vi "(150M)art联动采集V4.9(新增双行扫描模块).vi"() -> ()   [LabVIEW 2016]
uses:
  <vilib>/Utility/file.llb/Write Delimited Spreadsheet (DBL).vi
  E:/PCI8552B/Driver/INF/Win32&Win64/amd64/PCI8552B_32.dll
  <vilib>/Utility/file.llb/Read Delimited Spreadsheet (I64).vi
  <vilib>/Instr/_visa.llb/VISA Configure Serial Port (Instr).vi
panel:
  out "量程选择":i32(ring)=1 items=["±1000mV", "±5000mV"]
  out "待读取数据长度":i32
  in  "单行？":enum32{"单行", "双行"}(radio)
  in  "色码表导入":path=path "C:/Users/H301/Desktop/art闭环扫描程序/色码表/色码表（彩色2）.txt" caption="（色码表导入）"
  out "水平进度条":u8(slide) scale=0.0..100.0
  out "x+y 3":dbl=3.0
  in  "分层图查看":bool
  in  "hDevice 2":i32
  in  "逐行扫描":bool
  in  "定位模式":bool
  in  "X终点":dbl
  in  "Y终点":dbl
  in  "高级设置":bool
  in  "Y轴回零速度":dbl=15000.0
  in  "X轴回零速度":dbl=15000.0
  in  "细分设置":dbl=8.0
  in  "等待时间":u32=40
  in  "文件保存":path=path "C:/Users/H301/Desktop/art采集实验数据" caption="保存路径"
  out "已用时（s）":dbl format="%<%H:%M:%S>t"
  out "error out":errorcluster caption="错误输出"
  in  "退出扫描(Esc)":bool
  in  "N_Length":i32=8000000
  out "M_Length":i32
  out "hDevice":i32=241832032
  out "毫秒计时值":u32=3586537
  out "数组":dbl[][](array[numeric])=[[58819.77200735986, 88200.32943600747]]
  out "强度图":dbl[][](graph)=[[58819.77200735986, 88200.32943600747]]
  out "judge":dbl
  out "Xloop":dbl
  out "幅频谱":dbl[](graph)
  out "时域谱":dbl[](graph)
  out "错误输出":errorcluster
  in  "启动":bool
  in  "逐点扫描":bool
  in  "X归零":bool
  in  "Y归零":bool
  in  "Y起点":dbl
  in  "Y轴速度":dbl=9000.0
  in  "X轴速度":dbl=9000.0
  out "电机状态":bool
  in  "电机端口":refnum<visa-resource-name>="COM6"
  out "Yloop":dbl=1.0
  out "X扫描范围":dbl=150.0
  out "Y扫描范围":dbl=75.0
  out "Y序":i32
  in  "X起点":dbl
  out "Y(mm)":dbl
  out "x+y 2":dbl=3.0
  in  "Y:":dbl=1.0
  in  "精度":dbl=0.001
  in  "电机急停":bool
  out "X（mm）":dbl
  out "x+y":dbl=1.0
  in  "X:":dbl=1.0
  # "实时坐标"
  # "时域谱"
  # "频域谱"
  # "归零"
  # "扫描区域"
  # "扫描步进(mm)"
  # "X:"
  # "~"
  # "Y:"
  # "~"
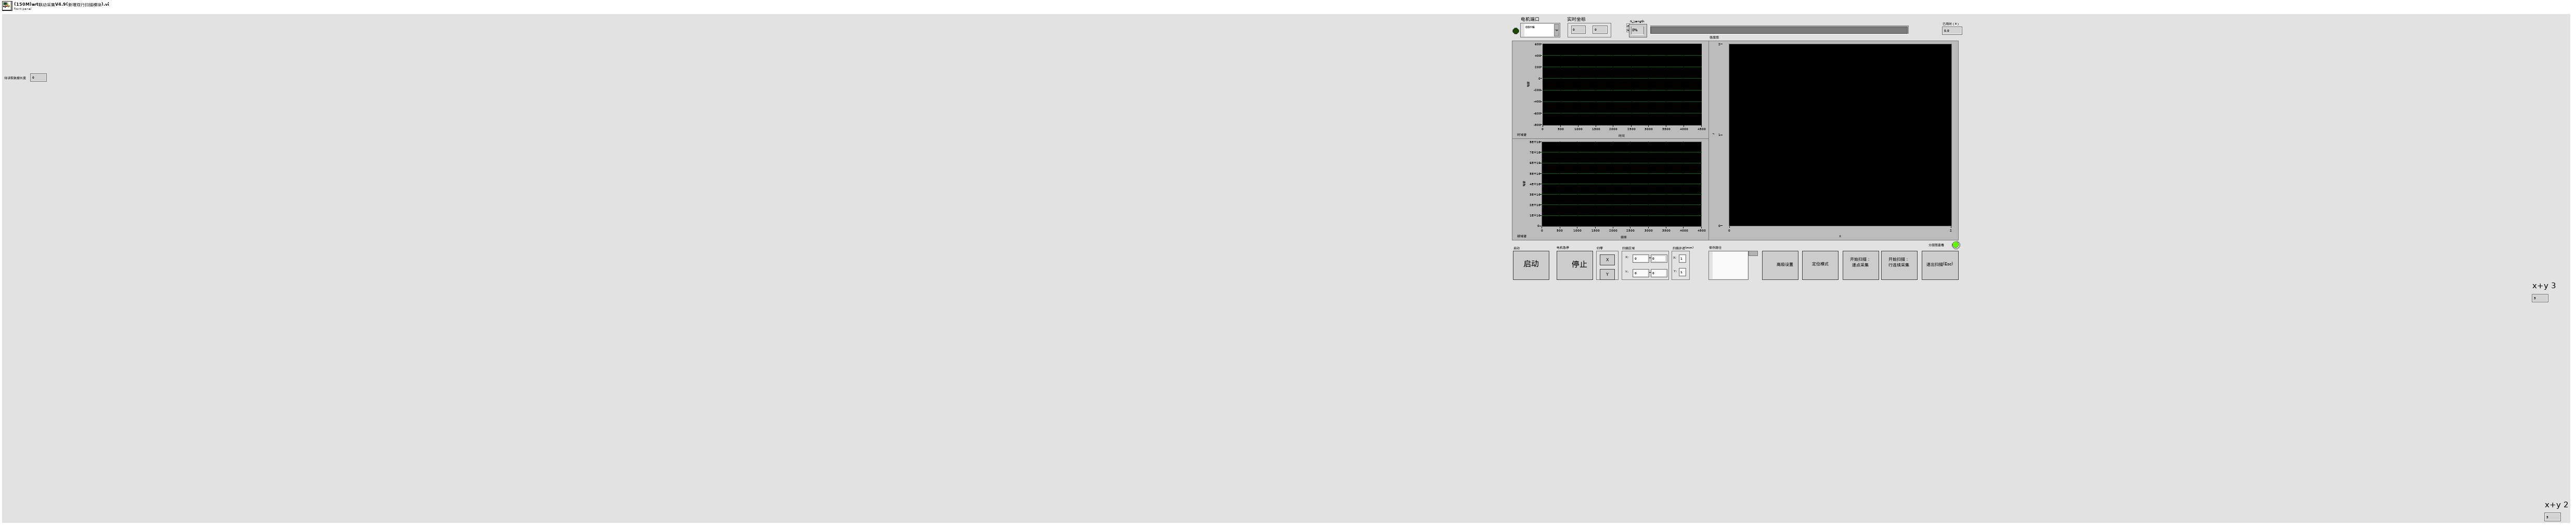
[diagram p1: front panel]
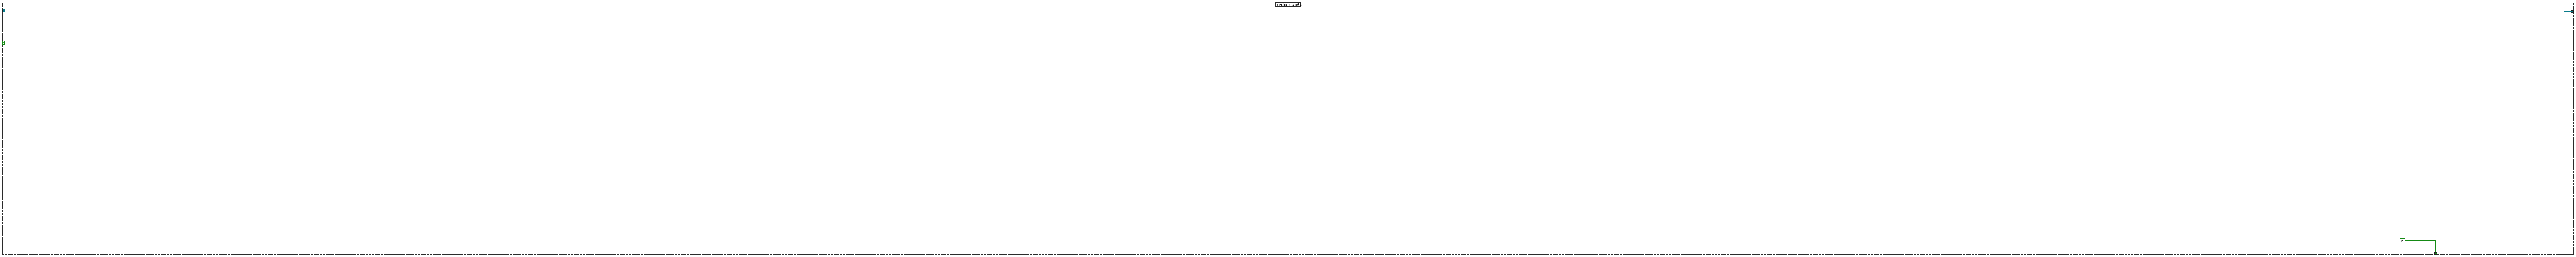
[diagram p3: hidden frame]
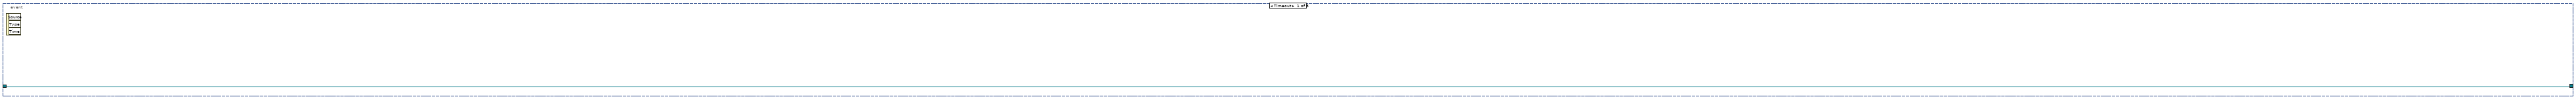
[diagram p4: hidden frame]
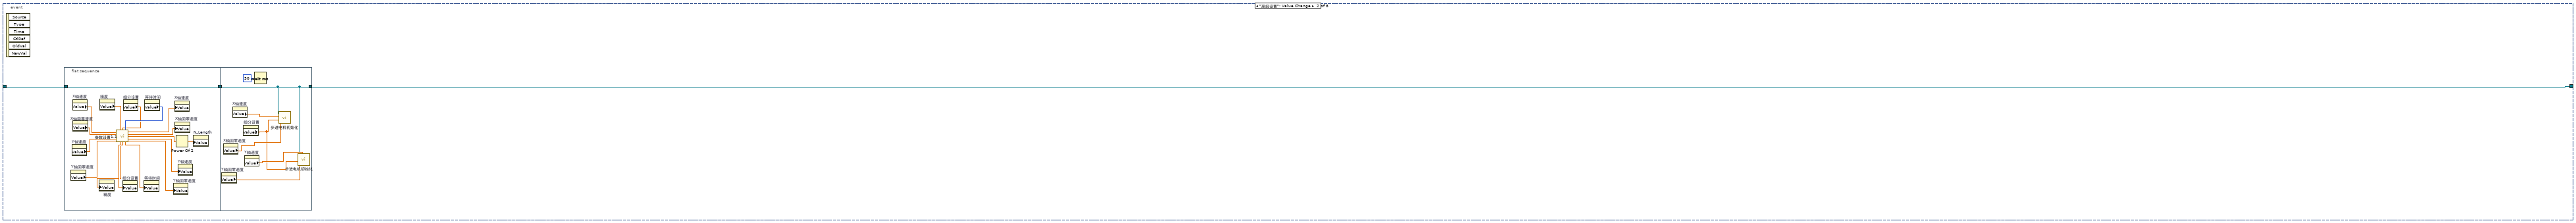
[diagram p5: hidden frame]
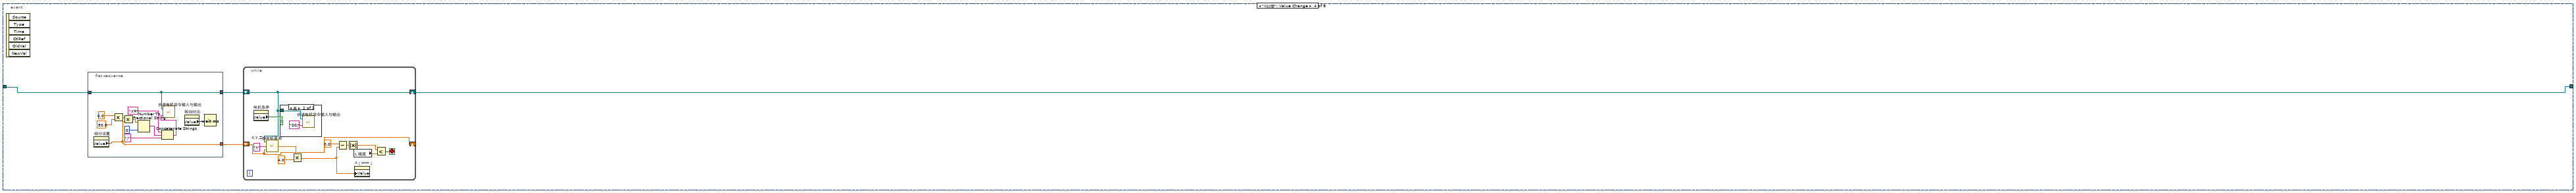
[diagram p6: hidden frame]
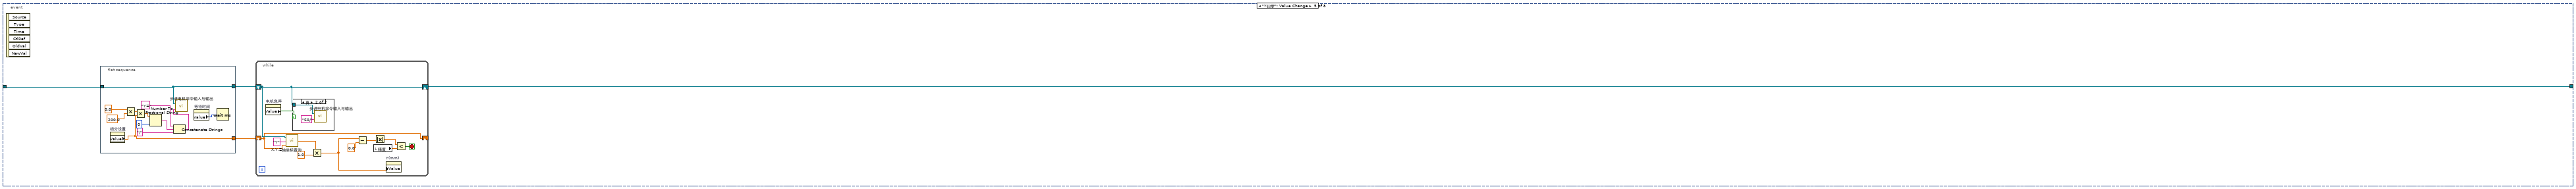
[diagram p8: hidden frame]
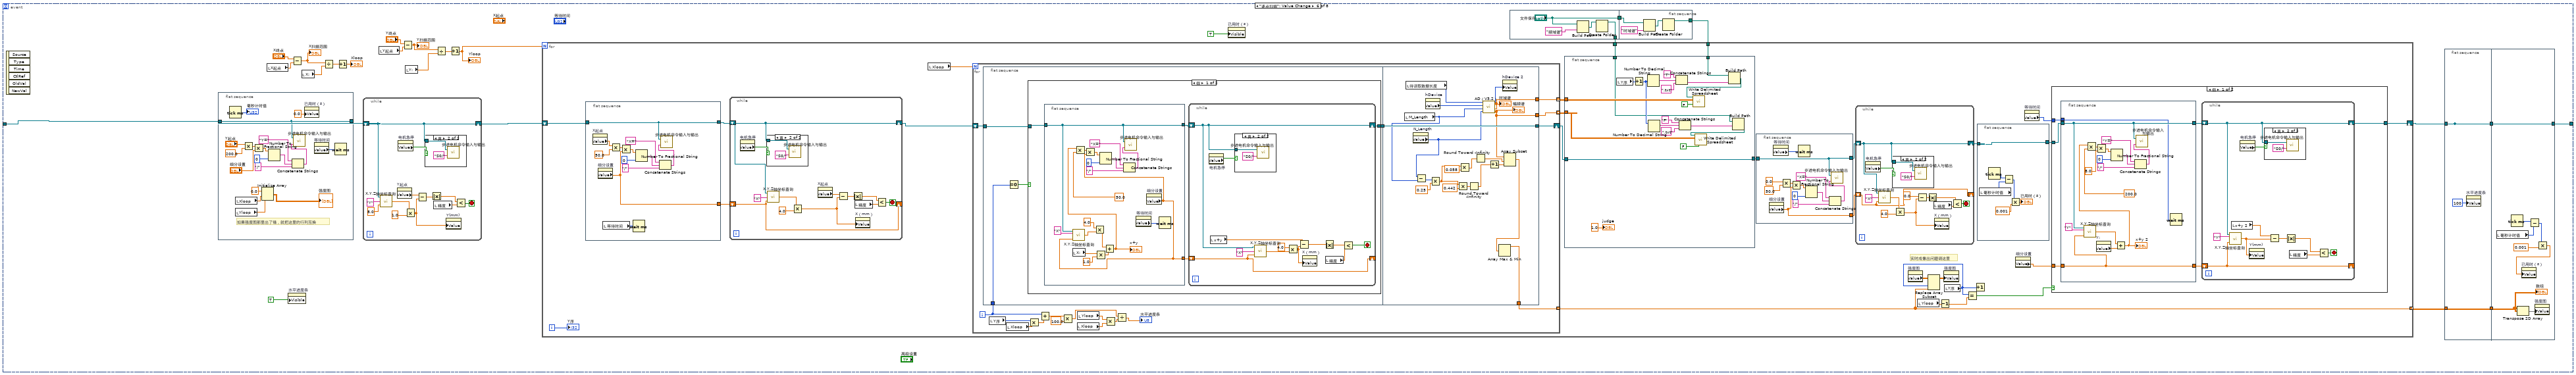
[diagram p10: hidden frame]
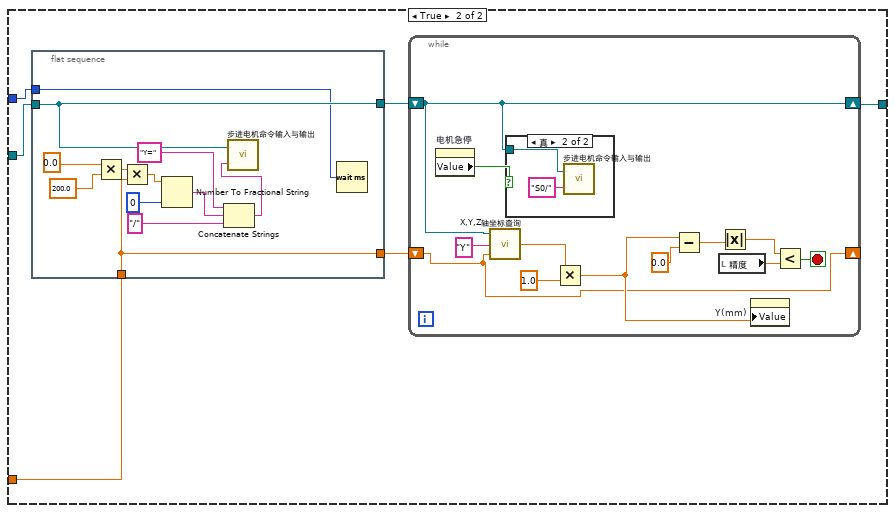
[diagram p15: hidden frame]
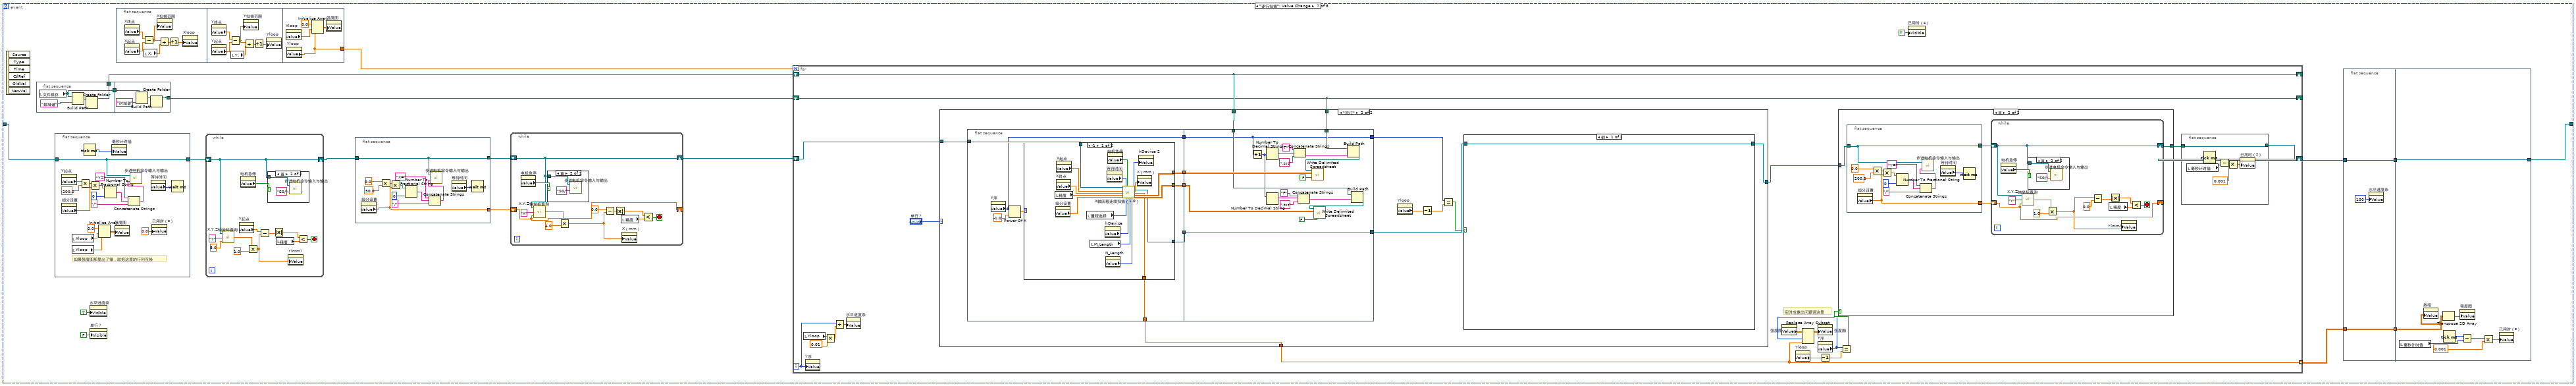
[diagram p19: hidden frame]
diagram:
  n1 = call-poly <vilib>:"Read Delimited Spreadsheet.vi"("file path (dialog if empty)"="色码表导入") -> ("first row"=w2:i64[])  [unwired: 9 in, 5 out]
  n2 = property on="强度图" class="IntGraph (严格)"("Color Table"=w2) -> ()  [unwired: 2 in, 2 out]
  n3 = property on="水平进度条" class="Slide (严格)"("Visible"=FALSE ("可见")) -> ()  [unwired: 2 in, 2 out]
  n4 = property on="单行？" class="RadioBtnsControl (严格)"("Visible"=TRUE ("可见")) -> ()  [unwired: 2 in, 2 out]
  n5 = while {
    stop <- w8 stop-if-true
    n6 = case shown="假" "启动" {
      tunnel: [FALSE ("ESC") w48] -> w8
      frame False {
      }
      frame True {
        w15 = 0  # M
        w25 = 1 items=["交流", "直流"]  # 耦合
        w23 = 1 items=["±1000mV", "±5000mV"]  # 量程选择
        w27 = TRUE  # 通道使能
        w21 = 20000000  # 采集频率
        w32 = 0 items=["中间触发", "后触发", "预触发", "硬件延时触发"]  # 触发模式
        w30 = 0 items=["通道0", "通道1"]  # ATR通道
        w41 = 0 items=["软件触发", "DTR作为触发源", "ATR作为触发源", "Trigger信号触发"]  # 触发源
        w40 = 0 items=["下降沿触发", "上升沿触发", "上下边沿均触发", ""]  # 触发方向
        w39 = 0  # 触发电平
        w24 = 1  # 触发次数
        w37 = 0 items=["TRIG0", "TRIG1", "TRIG2", "TRIG3"]  # 时钟输入输出源
        w38 = 0 items=["内时钟源", "主卡10M时钟源", "外部时钟"]  # 时钟源选择
        w61 = u16 0 items=["无", "XON/XOFF", "RTS/CTS", "XON/XOFF & RTS/CTS", "DTR/DSR", "XON/XOFF & DTR/DSR"] ("flow control (0:none)")
        w62 = u16 10 items=["1.0"=10, "1.5"=15, "2.0"=20] ("stop bits (10: 1 bit)")
        n7 = Boolean To (0,1)(Boolean=w27) -> (0, 1=w34:i16)
        n8 = Boolean To (0,1)(Boolean=FALSE ("主设备使能")) -> (0, 1=w35:i16)
        n9 = To Long Integer(number=w34) -> (32bit integer=w26:i32)
        n10 = To Long Integer(number=w35) -> (32bit integer=w36:i32)
        n11 = call-poly "VISA Configure Serial Port"("VISA resource name"="电机端口", "baud rate (9600)"=u32 9600, "data bits (8)"=u16 8, "parity (0:none)"=enum16{"None", "Odd", "Even", "Mark", "Space"}."None", "stop bits (10: 1 bit)"=w62, "flow control (0:none)"=w61) -> ("VISA resource name out"=w53:refnum<visa-resource-name>, "error out"=→"error out":errorcluster)  [unwired: 1 in, 7 out]
        n12 = Build Array(w26, w26) -> (w22:i32[])
        n13 = Build Array(w23, w23) -> (w31:i32[])
        n14 = Build Array(w25, w25) -> (w42:i32[])
        n15 = property on="细分设置" class="DigNum (严格)"() -> ("Value"=w47:dbl)  [unwired: 2 in, 2 out]
        n16 = Add Array Elements(numeric array=w22) -> (sum=w17:i32)
        n17 = Build Array (concatenate)(w22, w21, w31, w42, w15, "N_Length", w32, w30, w41, w40, w39, w24, w38, w36, w37) -> (w33:i32[])
        n18 = call "步进电机初始化.vi"("回零速度"="X轴回零速度", "细分设置"=w47, "X轴速度"="X轴速度", "串口通信端口"=w53) -> ()  [unwired: 2 in, 1 out]
        n19 = dll-call lib="E:/PCI8552B/Driver/INF/Win32&Win64/amd64/PCI8552B_32.dll" fn="PCI8552B_CreateDevice" label="CreateDevice"("DeviceLgcID"=0) -> ("返回类型"=w28:i32)  [unwired: 4 in, 2 out]
        n20 = call "步进电机初始化.vi"("Y轴速度"="Y轴速度", "回零速度"="Y轴回零速度", "细分设置"=w47, "串口通信端口"=w53) -> ()  [unwired: 2 in, 1 out]
        n21 = call "步进电机命令输入与输出.vi"("输入字符串"="?R/", "串口通信端口"=w53) -> ("返回字符串"=w58:string)
        n22 = dll-call lib="E:/PCI8552B/Driver/INF/Win32&Win64/amd64/PCI8552B_32.dll" fn="PCI8552B_InitDeviceAD" label="InitDeviceAD"("hDevice"=w28, "pADPara"=w33) -> ("hDevice"=→"hDevice":i32)  [unwired: 5 in, 2 out]
        n23 = Add(x=w15, y="N_Length") -> (x+y=w18:i32)
        n24 = String Subset(string=w58, offset (0)=0 ("偏移量(0)"), length (rest)=2 ("长度（剩余）")) -> (substring=w55:string)
        n25 = Multiply(x=w17, y=w18) -> (x*y=w20:i32)
        n26 = Equal?(x=w55, y="OK") -> (x = y?=w52:bool)
        "电机状态" <- w52
        n27 = Multiply(x=w20, y=w24) -> (x*y=→"待读取数据长度":i32)
        n28 = case shown="真" w52 {
          tunnel: w53 -> [w68 w71]
          tunnel: [w68 w69] -> w49
          tunnel: [FALSE ("ESC") w70] -> w48
          frame False {
          }
          frame True {
            n29 = while {
              tunnel: ["退出扫描(Esc)"] -> w70
              shift-right: [w75] -> w69
              shift-left: w71 -> [w80]
              stop <- "退出扫描(Esc)" stop-if-true
              n30 = property on="水平进度条" class="Slide (严格)"("Visible"=FALSE ("可见")) -> ()  [unwired: 2 in, 2 out]
              n31 = property on="高级设置" class="Bool"("Visible"=TRUE ("可见")) -> ()  [unwired: 2 in, 2 out]
              n32 = property on="定位模式" class="Bool"("Visible"=TRUE ("可见")) -> ()  [unwired: 2 in, 2 out]
              n33 = property on="水平进度条" class="Slide (严格)"("Value"=u8 0 ("水平进度条")) -> ()  [unwired: 2 in, 2 out]
              n34 = property on="单行？" class="RadioBtnsControl (严格)"("Visible"=TRUE ("可见")) -> ()  [unwired: 2 in, 2 out]
              n35 = event shown="[2] \"定位模式\": 值改变" {
                selector: _ -> [_ _ _ _ _ _ _ _]
                dyn-events: _ -> [_ _ _ _ _ _ _ _]
                timeout: 1 -> [_ _ _ _ _ _ _ _]
                tunnel: w80 -> [w81 w84 w118 w122 w152 w203 w517 w882]
                tunnel: [w81 w83 w117 w120 w150 w198 w519 w881] -> w75
                event Timeout {
                  n36 = event-data() -> ()  [unwired: 1 in, 3 out]
                }
                event "高级设置": Value Change {
                  n37 = event-data() -> ()  [unwired: 1 in, 6 out]
                  n38 = flat-sequence {
                    tunnel: w84 -> [w87]
                    tunnel: [w87] -> w82
                    tunnel: [w103] -> w83
                    tunnel: w82 -> [w103]
                    frame #0 {
                      n39 = property on="Y轴回零速度" class="DigNum (严格)"() -> ("Value"=w91:dbl)  [unwired: 2 in, 2 out]
                      n40 = property on="Y轴速度" class="DigNum (严格)"() -> ("Value"=w90:dbl)  [unwired: 2 in, 2 out]
                      n41 = property on="X轴速度" class="DigNum (严格)"() -> ("Value"=w88:dbl)  [unwired: 2 in, 2 out]
                      n42 = property on="X轴回零速度" class="DigNum (严格)"() -> ("Value"=w89:dbl)  [unwired: 2 in, 2 out]
                      n43 = property on="精度" class="DigNum (严格)"() -> ("Value"=w95:dbl)  [unwired: 2 in, 2 out]
                      n44 = property on="细分设置" class="DigNum (严格)"() -> ("Value"=w96:dbl)  [unwired: 2 in, 2 out]
                      n45 = property on="等待时间" class="DigNum (严格)"() -> ("Value"=w97:u32)  [unwired: 2 in, 2 out]
                      n46 = call "参数设置1.1.vi"("X轴速度"=w88, "精度"=w95, "细分设置"=w96, "等待时间"=w97, "X轴回零速度"=w89, "Y轴速度"=w90, "Y轴回零速度"=w91) -> ("X轴速度"=w98:dbl, "X轴回零速度"=w99:dbl, "采样阶"=w85:dbl, "Y轴速度"=w100:dbl, "精度"=w92:dbl, "细分设置"=w93:dbl, "等待时间"=w94:dbl, "Y轴回零速度"=w101:dbl)  [unwired: 1 in]
                      n47 = property on="精度" class="DigNum (严格)"("Value"=w92) -> ()  [unwired: 2 in, 2 out]
                      n48 = property on="细分设置" class="DigNum (严格)"("Value"=w93) -> ()  [unwired: 2 in, 2 out]
                      n49 = property on="等待时间" class="DigNum (严格)"("Value"=w94) -> ()  [unwired: 2 in, 2 out]
                      n50 = property on="Y轴回零速度" class="DigNum (严格)"("Value"=w101) -> ()  [unwired: 2 in, 2 out]
                      n51 = property on="X轴速度" class="DigNum (严格)"("Value"=w98) -> ()  [unwired: 2 in, 2 out]
                      n52 = property on="X轴回零速度" class="DigNum (严格)"("Value"=w99) -> ()  [unwired: 2 in, 2 out]
                      n53 = Power Of 2(x=w85) -> (2^x=w86:dbl)
                      n54 = property on="Y轴速度" class="DigNum (严格)"("Value"=w100) -> ()  [unwired: 2 in, 2 out]
                      n55 = property on="N_Length" class="DigNum (严格)"("Value"=w86) -> ()  [unwired: 2 in, 2 out]
                    }
                    frame #1 {
                      n56 = property on="Y轴回零速度" class="DigNum (严格)"() -> ("Value"=w107:dbl)  [unwired: 2 in, 2 out]
                      n57 = property on="X轴回零速度" class="DigNum (严格)"() -> ("Value"=w106:dbl)  [unwired: 2 in, 2 out]
                      n58 = property on="X轴速度" class="DigNum (严格)"() -> ("Value"=w105:dbl)  [unwired: 2 in, 2 out]
                      n59 = property on="细分设置" class="DigNum (严格)"() -> ("Value"=w104:dbl)  [unwired: 2 in, 2 out]
                      n60 = property on="Y轴速度" class="DigNum (严格)"() -> ("Value"=w108:dbl)  [unwired: 2 in, 2 out]
                      n61 = Wait (ms)(milliseconds to wait=u32 50 ("等待时间（毫秒）")) -> ()  [unwired: 1 out]
                      n62 = call "步进电机初始化.vi"("回零速度"=w106, "细分设置"=w104, "X轴速度"=w105, "串口通信端口"=w103) -> ()  [unwired: 2 in, 1 out]
                      n63 = call "步进电机初始化.vi"("Y轴速度"=w108, "回零速度"=w107, "细分设置"=w104, "串口通信端口"=w103) -> ()  [unwired: 2 in, 1 out]
                    }
                  }
                }
                event "定位模式": Value Change {
                  n64 = event-data() -> ()  [unwired: 1 in, 6 out]
                  n65 = local read "待读取数据长度"() -> (w114:i32)
                  n66 = local read "M_Length"() -> (w112:i32)
                  n67 = local read "量程选择"() -> (w109:i32)
                  n68 = property on="hDevice" class="DigNum (严格)"() -> ("Value"=w113:i32)  [unwired: 2 in, 2 out]
                  n69 = property on="N_Length" class="DigNum (严格)"() -> ("Value"=w111:i32)  [unwired: 2 in, 2 out]
                  n70 = call "电机定位1.1（只处理采集卡）.vi"("VISA I"=w118, "pulDDR2Length"=w114, "量程选择"=w109, "hDevice"=w113, "M-length"=w112, "N-length"=w111) -> ("hDevice out"=w110:i32, "VISA O"=w117:refnum<visa-resource-name>, "X"=w116:dbl, "Y"=w115:dbl)  [unwired: 10 in]
                  n71 = property on="hDevice 2" class="DigNum (严格)"("Value"=w110) -> ()  [unwired: 2 in, 2 out]
                  n72 = property on="X（mm）" class="DigNum (严格)"("Value"=w116) -> ()  [unwired: 2 in, 2 out]
                  n73 = property on="Y(mm)" class="DigNum (严格)"("Value"=w115) -> ()  [unwired: 2 in, 2 out]
                }
                event "X归零": Value Change {
                  n74 = event-data() -> ()  [unwired: 1 in, 6 out]
                  n75 = flat-sequence {
                    tunnel: w122 -> [w126]
                    tunnel: [w126] -> w121
                    tunnel: [w123] -> w119
                    frame #0 {
                      n76 = property on="细分设置" class="DigNum (严格)"() -> ("Value"=w123:dbl)  [unwired: 2 in, 2 out]
                      n77 = Multiply(x=0.0, y=50.0) -> (x*y=w129:dbl)
                      n78 = Multiply(x=w129, y=w123) -> (x*y=w134:dbl)
                      n79 = Number To Fractional String(number=w134, precision (6)=i16 0 ("精度(6)")) -> (F-format string=w132:string)  [unwired: 2 out]
                      n80 = Concatenate Strings("X=" ("字符串"), w132, "/" ("字符串")) -> (w127:string)
                      n81 = call "步进电机命令输入与输出.vi"("输入字符串"=w127, "串口通信端口"=w126) -> ()  [unwired: 1 out]
                      n82 = property on="等待时间" class="DigNum (严格)"() -> ("Value"=w124:u32)  [unwired: 2 in, 2 out]
                      n83 = Wait (ms)(milliseconds to wait=w124) -> ()  [unwired: 1 out]
                    }
                  }
                  n84 = while {
                    shift-right: [w136] -> w120
                    shift-left: w121 -> [w136]
                    shift-right: [w135] -> _
                    shift-left: w119 -> [w135]
                    stop <- w142 stop-if-true
                    n85 = property on="电机急停" class="Bool (严格)"() -> ("Value"=w143:bool)  [unwired: 2 in, 2 out]
                    n86 = call "X,Y,Z轴坐标查询.vi"("细分设置"=w135, "查询坐标轴"="X", "串口通信端口"=w136) -> ("坐标(mm)"=w144:dbl)
                    n87 = case shown="真" w143 {
                      tunnel: w136 -> [_ w147]
                      frame False {
                      }
                      frame True {
                        n88 = call "步进电机命令输入与输出.vi"("输入字符串"="S0/", "串口通信端口"=w147) -> ()  [unwired: 1 out]
                      }
                    }
                    n89 = Multiply(x=w144, y=4.0 ("x")) -> (x*y=w140:dbl)
                    n90 = Subtract(x=0.0, y=w140) -> (x-y=w139:dbl)
                    n91 = Absolute Value(x=w139) -> (abs(x)=w138:dbl)
                    n92 = local read "精度"() -> (w141:dbl)
                    n93 = property on="X（mm）" class="DigNum (严格)"("Value"=w140) -> ()  [unwired: 2 in, 2 out]
                    n94 = Less?(x=w138, y=w141) -> (x < y?=w142:bool)
                  }
                }
                event "Y归零": Value Change {
                  n95 = event-data() -> ()  [unwired: 1 in, 6 out]
                  n96 = flat-sequence {
                    tunnel: w152 -> [w156]
                    tunnel: [w156] -> w151
                    tunnel: [w153] -> w149
                    frame #0 {
                      n97 = property on="细分设置" class="DigNum (严格)"() -> ("Value"=w153:dbl)  [unwired: 2 in, 2 out]
                      n98 = Multiply(x=0.0, y=200.0) -> (x*y=w159:dbl)
                      n99 = Multiply(x=w159, y=w153) -> (x*y=w164:dbl)
                      n100 = Number To Fractional String(number=w164, precision (6)=i16 0 ("精度(6)")) -> (F-format string=w162:string)  [unwired: 2 out]
                      n101 = Concatenate Strings("Y=" ("字符串"), w162, "/" ("字符串")) -> (w157:string)
                      n102 = call "步进电机命令输入与输出.vi"("输入字符串"=w157, "串口通信端口"=w156) -> ()  [unwired: 1 out]
                      n103 = property on="等待时间" class="DigNum (严格)"() -> ("Value"=w154:u32)  [unwired: 2 in, 2 out]
                      n104 = Wait (ms)(milliseconds to wait=w154) -> ()  [unwired: 1 out]
                    }
                  }
                  n105 = while {
                    shift-right: [w166] -> w150
                    shift-left: w151 -> [w166]
                    shift-right: [w165] -> _
                    shift-left: w149 -> [w165]
                    stop <- w172 stop-if-true
                    n106 = property on="电机急停" class="Bool (严格)"() -> ("Value"=w173:bool)  [unwired: 2 in, 2 out]
                    n107 = call "X,Y,Z轴坐标查询.vi"("细分设置"=w165, "查询坐标轴"="Y", "串口通信端口"=w166) -> ("坐标(mm)"=w174:dbl)
                    n108 = case shown="真" w173 {
                      tunnel: w166 -> [_ w177]
                      frame False {
                      }
                      frame True {
                        n109 = call "步进电机命令输入与输出.vi"("输入字符串"="S0/", "串口通信端口"=w177) -> ()  [unwired: 1 out]
                      }
                    }
                    n110 = Multiply(x=w174, y=1.0 ("x")) -> (x*y=w170:dbl)
                    n111 = Subtract(x=w170, y=0.0 ("x")) -> (x-y=w168:dbl)
                    n112 = local read "精度"() -> (w171:dbl)
                    n113 = Absolute Value(x=w168) -> (abs(x)=w167:dbl)
                    n114 = property on="Y(mm)" class="DigNum (严格)"("Value"=w170) -> ()  [unwired: 2 in, 2 out]
                    n115 = Less?(x=w167, y=w171) -> (x < y?=w172:bool)
                  }
                }
                event "逐点扫描": Value Change {
                  n116 = event-data() -> ()  [unwired: 1 in, 6 out]
                  n117 = flat-sequence {
                    tunnel: w203 -> [w232]
                    tunnel: [w232] -> w194
                    frame #0 {
                      # "如果强度图那里出了错，就把这里的行列互换"
                      n118 = Tick Count (ms)() -> (millisecond timer value=→"毫秒计时值":u32)
                      n119 = local read "Xloop"() -> (w227:dbl)
                      n120 = local read "Yloop"() -> (w226:dbl)
                      n121 = Multiply(x="Y起点", y=200.0) -> (x*y=w235:dbl)
                      n122 = Multiply(x=w235, y="细分设置") -> (x*y=w240:dbl)
                      n123 = Initialize Array(0.0 ("元素"), w227, w226) -> (→"强度图":dbl[][])
                      n124 = Number To Fractional String(number=w240, precision (6)=i16 0 ("精度(6)")) -> (F-format string=w238:string)  [unwired: 2 out]
                      n125 = Concatenate Strings("Y=" ("字符串"), w238, "/" ("字符串")) -> (w233:string)
                      n126 = call "步进电机命令输入与输出.vi"("输入字符串"=w233, "串口通信端口"=w232) -> ()  [unwired: 1 out]
                      n127 = property on="已用时（s）" class="DigNum (严格)"("Value"=0.0 ("已用时（s）")) -> ()  [unwired: 2 in, 2 out]
                      n128 = property on="等待时间" class="DigNum (严格)"() -> ("Value"=w224:u32)  [unwired: 2 in, 2 out]
                      n129 = Wait (ms)(milliseconds to wait=w224) -> ()  [unwired: 1 out]
                    }
                  }
                  n130 = local read "X起点"() -> (w190:dbl)
                  n131 = property on="水平进度条" class="Slide (严格)"("Visible"=TRUE ("可见")) -> ()  [unwired: 2 in, 2 out]
                  n132 = Subtract(x="X终点", y=w190) -> (x-y=w189:dbl)
                  "X扫描范围" <- w189
                  n133 = local read "X:"() -> (w197:dbl)
                  n134 = Divide(x=w189, y=w197) -> (x/y=w195:dbl)
                  n135 = Increment(x=w195) -> (x+1=→"Xloop":dbl)
                  n136 = while {
                    shift-right: [w241] -> w186
                    shift-left: w194 -> [w241]
                    stop <- w246 stop-if-true
                    n137 = call "X,Y,Z轴坐标查询.vi"("细分设置"=8.0, "查询坐标轴"="Y", "串口通信端口"=w241) -> ("坐标(mm)"=w248:dbl)
                    n138 = property on="Y起点" class="DigNum (严格)"() -> ("Value"=w250:dbl)  [unwired: 2 in, 2 out]
                    n139 = property on="电机急停" class="Bool (严格)"() -> ("Value"=w247:bool)  [unwired: 2 in, 2 out]
                    n140 = Multiply(x=w248, y=1.0 ("x")) -> (x*y=w244:dbl)
                    n141 = Subtract(x=w250, y=w244) -> (x-y=w243:dbl)
                    n142 = case shown="真" w247 {
                      tunnel: w241 -> [_ w253]
                      frame False {
                      }
                      frame True {
                        n143 = call "步进电机命令输入与输出.vi"("输入字符串"="S0/", "串口通信端口"=w253) -> ()  [unwired: 1 out]
                      }
                    }
                    n144 = Absolute Value(x=w243) -> (abs(x)=w242:dbl)
                    n145 = local read "精度"() -> (w245:dbl)
                    n146 = property on="Y(mm)" class="DigNum (严格)"("Value"=w244) -> ()  [unwired: 2 in, 2 out]
                    n147 = Less?(x=w242, y=w245) -> (x < y?=w246:bool)
                  }
                  n148 = local read "Y起点"() -> (w192:dbl)
                  n149 = Subtract(x="Y终点", y=w192) -> (x-y=w188:dbl)
                  "Y扫描范围" <- w188
                  n150 = local read "Y:"() -> (w202:dbl)
                  n151 = Divide(x=w188, y=w202) -> (x/y=w201:dbl)
                  n152 = Increment(x=w201) -> (x+1=w200:dbl)
                  "Yloop" <- w200
                  n153 = for {
                    N: w200 -> [_]
                    shift-right: [w278] -> w179
                    shift-left: w186 -> [w259]
                    tunnel: [w261] -> w199 mode=indexing
                    tunnel: w184 -> [w265]
                    tunnel: w187 -> [w264]
                    i -> [w279]
                    # "实时成像出问题调这里"
                    n154 = flat-sequence {
                      tunnel: w259 -> [w336]
                      tunnel: [w336] -> w277
                      tunnel: [w335] -> w269
                      frame #0 {
                        n155 = property on="X起点" class="DigNum (严格)"() -> ("Value"=w333:dbl)  [unwired: 2 in, 2 out]
                        n156 = property on="细分设置" class="DigNum (严格)"() -> ("Value"=w335:dbl)  [unwired: 2 in, 2 out]
                        n157 = local read "等待时间"() -> (w334:u32)
                        n158 = Multiply(x=w333, y=50.0) -> (x*y=w339:dbl)
                        n159 = Multiply(x=w339, y=w335) -> (x*y=w344:dbl)
                        n160 = Wait (ms)(milliseconds to wait=w334) -> ()  [unwired: 1 out]
                        n161 = Number To Fractional String(number=w344, precision (6)=i16 0 ("精度(6)")) -> (F-format string=w342:string)  [unwired: 2 out]
                        n162 = Concatenate Strings("X=" ("字符串"), w342, "/" ("字符串")) -> (w337:string)
                        n163 = call "步进电机命令输入与输出.vi"("输入字符串"=w337, "串口通信端口"=w336) -> ()  [unwired: 1 out]
                      }
                    }
                    n164 = while {
                      shift-right: [w346] -> w257
                      shift-left: w277 -> [w346]
                      shift-right: [w345] -> _
                      shift-left: w269 -> [w345]
                      stop <- w351 stop-if-true
                      n165 = property on="电机急停" class="Bool (严格)"() -> ("Value"=w352:bool)  [unwired: 2 in, 2 out]
                      n166 = case shown="真" w352 {
                        tunnel: w346 -> [_ w357]
                        frame False {
                        }
                        frame True {
                          n167 = call "步进电机命令输入与输出.vi"("输入字符串"="S0/", "串口通信端口"=w357) -> ()  [unwired: 1 out]
                        }
                      }
                      n168 = call "X,Y,Z轴坐标查询.vi"("细分设置"=w345, "查询坐标轴"="X", "串口通信端口"=w346) -> ("坐标(mm)"=w353:dbl)
                      n169 = Multiply(x=w353, y=4.0 ("x")) -> (x*y=w349:dbl)
                      n170 = property on="X起点" class="DigNum (严格)"() -> ("Value"=w355:dbl)  [unwired: 2 in, 2 out]
                      n171 = Subtract(x=w355, y=w349) -> (x-y=w348:dbl)
                      n172 = Absolute Value(x=w348) -> (abs(x)=w347:dbl)
                      n173 = local read "精度"() -> (w350:dbl)
                      n174 = property on="X（mm）" class="DigNum (严格)"("Value"=w349) -> ()  [unwired: 2 in, 2 out]
                      n175 = Less?(x=w347, y=w350) -> (x < y?=w351:bool)
                    }
                    n176 = local read "Xloop"() -> (w270:dbl)
                    n177 = for {
                      N: w270 -> [_]
                      shift-right: [w440] -> w258
                      shift-left: w257 -> [w436]
                      tunnel: [w439] -> w276 mode=indexing
                      tunnel: [w438] -> w275 mode=indexing
                      tunnel: [w437] -> w261 mode=indexing
                      i -> [w428]
                      n178 = flat-sequence {
                        tunnel: w436 -> [w445]
                        tunnel: [w444] -> w441
                        tunnel: w428 -> [w442]
                        tunnel: [w503] -> w440
                        tunnel: w441 -> [w503]
                        tunnel: [w502] -> w439
                        tunnel: [w501] -> w438
                        tunnel: [w499] -> w437
                        frame #0 {
                          n179 = Equal To 0?(x=w442) -> (x = 0?=w443:bool)
                          n180 = case shown="假" w443 {
                            tunnel: w445 -> [w448 w483]
                            tunnel: [w447 w483] -> w444
                            frame False {
                              n181 = flat-sequence {
                                tunnel: w448 -> [w458]
                                tunnel: [w458] -> w449
                                tunnel: [w450] -> w446
                                frame #0 {
                                n182 = local read "X:"() -> (w452:dbl)
                                n183 = Multiply(x=w452, y=1.0 ("x")) -> (x*y=w457:dbl)
                                n184 = property on="等待时间" class="DigNum (严格)"() -> ("Value"=w451:u32)  [unwired: 2 in, 2 out]
                                n185 = property on="细分设置" class="DigNum (严格)"() -> ("Value"=w450:dbl)  [unwired: 2 in, 2 out]
                                n186 = call "X,Y,Z轴坐标查询.vi"("细分设置"=w450, "查询坐标轴"="X", "串口通信端口"=w458) -> ("坐标(mm)"=w454:dbl)
                                n187 = Multiply(x=4.0, y=w454) -> (x*y=w453:dbl)
                                n188 = Add(x=w453, y=w457) -> (x+y=w460:dbl)
                                "x+y" <- w460
                                n189 = Multiply(x=w460, y=50.0) -> (x*y=w463:dbl)
                                n190 = Multiply(x=w463, y=w450) -> (x*y=w468:dbl)
                                n191 = Number To Fractional String(number=w468, precision (6)=i16 0 ("精度(6)")) -> (F-format string=w466:string)  [unwired: 2 out]
                                n192 = Concatenate Strings("X=" ("字符串"), w466, "/" ("字符串")) -> (w461:string)
                                n193 = call "步进电机命令输入与输出.vi"("输入字符串"=w461, "串口通信端口"=w458) -> ()  [unwired: 1 out]
                                n194 = Wait (ms)(milliseconds to wait=w451) -> ()  [unwired: 1 out]
                                }
                              }
                              n195 = while {
                                shift-right: [w478] -> w447
                                shift-left: w449 -> [w478]
                                shift-right: [w469] -> _
                                shift-left: w446 -> [w469]
                                stop <- w477 stop-if-true
                                n196 = property on="电机急停" class="Bool (严格)"() -> ("Value"=w475:bool)  [unwired: 2 in, 2 out]
                                n197 = local read "x+y"() -> (w479:dbl)
                                n198 = case shown="真" w475 {
                                tunnel: w478 -> [_ w481]
                                frame False {
                                }
                                frame True {
                                n199 = call "步进电机命令输入与输出.vi"("输入字符串"="S0/", "串口通信端口"=w481) -> ()  [unwired: 1 out]
                                }
                                }
                                n200 = call "X,Y,Z轴坐标查询.vi"("细分设置"=w469, "查询坐标轴"="X", "串口通信端口"=w478) -> ("坐标(mm)"=w473:dbl)
                                n201 = Multiply(x=4.0, y=w473) -> (x*y=w472:dbl)
                                n202 = Subtract(x=w479, y=w472) -> (x-y=w471:dbl)
                                n203 = property on="X（mm）" class="DigNum (严格)"("Value"=w472) -> ()  [unwired: 2 in, 2 out]
                                n204 = Absolute Value(x=w471) -> (abs(x)=w470:dbl)
                                n205 = local read "精度"() -> (w474:dbl)
                                n206 = Less?(x=w470, y=w474) -> (x < y?=w477:bool)
                              }
                            }
                            frame True {
                            }
                          }
                        }
                        frame #1 {
                          n207 = local read "M_Length"() -> (w497:i32)
                          n208 = local read "待读取数据长度"() -> (w498:i32)
                          n209 = property on="N_Length" class="DigNum (严格)"() -> ("Value"=w486:i32)  [unwired: 2 in, 2 out]
                          n210 = Subtract(x=w486, y=w497) -> (x-y=w495:i32)
                          n211 = property on="hDevice" class="DigNum (严格)"() -> ("Value"=w484:i32)  [unwired: 2 in, 2 out]
                          n212 = Multiply(x=w495, y=0.25) -> (x*y=w488:dbl)
                          n213 = Multiply(x=w488, y=0.442) -> (x*y=w490:dbl)
                          n214 = Multiply(x=w488, y=0.058) -> (x*y=w492:dbl)
                          n215 = Round Toward -Infinity(1:w490) -> (0:w487:dbl)
                          n216 = Round Toward -Infinity(1:w492) -> (0:w491:dbl)
                          n217 = call "AD（V3.2）.vi"("N-length"=w486, "M-length"=w497, "hDevice"=w484, "待读取数据长度"=w498) -> ("幅频谱"=w501:dbl[], "时域谱"=w502:dbl[], "hDevice out"=w485:i32)  [unwired: 5 in]
                          "时域谱" <- w502
                          "幅频谱" <- w501
                          n218 = Increment(x=w487) -> (x+1=w494:dbl)
                          n219 = property on="hDevice 2" class="DigNum (严格)"("Value"=w485) -> ()  [unwired: 2 in, 2 out]
                          n220 = Array Subset(array=w501, index=w491, length=w494) -> (w500:dbl[])
                          n221 = Array Max & Min(array=w500) -> (max value=w499:dbl)  [unwired: 3 out]
                        }
                      }
                      n222 = local read "Y序"() -> (w430:i32)
                      n223 = local read "Xloop"() -> (w431:dbl)
                      n224 = Multiply(x=w430, y=w431) -> (x*y=w429:dbl)
                      n225 = Add(x=w428, y=w429) -> (x+y=w427:dbl)
                      n226 = Multiply(x=w427, y=100.0) -> (x*y=w425:dbl)
                      n227 = local read "Xloop"() -> (w435:dbl)
                      n228 = local read "Yloop"() -> (w434:dbl)
                      n229 = Multiply(x=w434, y=w435) -> (x*y=w433:dbl)
                      n230 = Divide(x=w425, y=w433) -> (x/y=→"水平进度条":dbl)
                    }
                    n231 = flat-sequence {
                      tunnel: w275 -> [w319]
                      tunnel: w276 -> [w327]
                      tunnel: w258 -> [w331]
                      tunnel: [w331] -> w271
                      tunnel: w265 -> [w314]
                      tunnel: w264 -> [w313]
                      frame #0 {
                        n232 = local read "Y序"() -> (w315:i32)
                        n233 = Increment(x=w315) -> (x+1=w316:i32)
                        n234 = Number To Decimal String(number=w316) -> (decimal integer string=w325:string)  [unwired: 1 in]
                        n235 = Number To Decimal String(number=w316) -> (decimal integer string=w324:string)  [unwired: 1 in]
                        n236 = Concatenate Strings("T" ("字符串"), w325, ".txt" ("字符串")) -> (w328:string)
                        n237 = Concatenate Strings("F" ("字符串"), w324, ".txt" ("字符串")) -> (w322:string)
                        n238 = Build Path(base path=w314, name or relative path=w328) -> (appended path=w330:path)
                        n239 = call-poly <vilib>:"Write Delimited Spreadsheet.vi"("file path (dialog if empty)"=w330, "2D data"=w327, "transpose? (no:F)"=FALSE) -> ()  [unwired: 11 in, 2 out]
                        n240 = Build Path(base path=w313, name or relative path=w322) -> (appended path=w320:path)
                        n241 = call-poly <vilib>:"Write Delimited Spreadsheet.vi"("file path (dialog if empty)"=w320, "2D data"=w319, "transpose? (no:F)"=FALSE) -> ()  [unwired: 11 in, 2 out]
                        "judge" <- 1.0
                      }
                    }
                    n242 = flat-sequence {
                      tunnel: w271 -> [w290]
                      tunnel: [w290] -> w272
                      tunnel: [w288] -> w268
                      frame #0 {
                        n243 = property on="细分设置" class="DigNum (严格)"() -> ("Value"=w288:dbl)  [unwired: 2 in, 2 out]
                        n244 = property on="等待时间" class="DigNum (严格)"() -> ("Value"=w287:u32)  [unwired: 2 in, 2 out]
                        n245 = Multiply(x=0.0, y=50.0) -> (x*y=w293:dbl)
                        n246 = Multiply(x=w293, y=w288) -> (x*y=w298:dbl)
                        n247 = Wait (ms)(milliseconds to wait=w287) -> ()  [unwired: 1 out]
                        n248 = Number To Fractional String(number=w298, precision (6)=i16 0 ("精度(6)")) -> (F-format string=w296:string)  [unwired: 2 out]
                        n249 = Concatenate Strings("X=" ("字符串"), w296, "/" ("字符串")) -> (w291:string)
                        n250 = call "步进电机命令输入与输出.vi"("输入字符串"=w291, "串口通信端口"=w290) -> ()  [unwired: 1 out]
                      }
                    }
                    n251 = while {
                      shift-right: [w300] -> w256
                      shift-left: w272 -> [w300]
                      shift-right: [w299] -> _
                      shift-left: w268 -> [w299]
                      stop <- w306 stop-if-true
                      n252 = property on="电机急停" class="Bool (严格)"() -> ("Value"=w307:bool)  [unwired: 2 in, 2 out]
                      n253 = call "X,Y,Z轴坐标查询.vi"("细分设置"=w299, "查询坐标轴"="X", "串口通信端口"=w300) -> ("坐标(mm)"=w308:dbl)
                      n254 = case shown="真" w307 {
                        tunnel: w300 -> [_ w311]
                        frame False {
                        }
                        frame True {
                          n255 = call "步进电机命令输入与输出.vi"("输入字符串"="S0/", "串口通信端口"=w311) -> ()  [unwired: 1 out]
                        }
                      }
                      n256 = Multiply(x=w308, y=4.0 ("x")) -> (x*y=w304:dbl)
                      n257 = Subtract(x=0.0, y=w304) -> (x-y=w303:dbl)
                      n258 = Absolute Value(x=w303) -> (abs(x)=w302:dbl)
                      n259 = local read "精度"() -> (w305:dbl)
                      n260 = property on="X（mm）" class="DigNum (严格)"("Value"=w304) -> ()  [unwired: 2 in, 2 out]
                      n261 = Less?(x=w302, y=w305) -> (x < y?=w306:bool)
                    }
                    n262 = property on="强度图" class="IntGraph (严格)"() -> ("Value"=w262:dbl[][])  [unwired: 2 in, 2 out]
                    n263 = local read "Yloop"() -> (w273:dbl)
                    n264 = Decrement(x=w273) -> (x-1=w274:dbl)
                    n265 = local read "Y序"() -> (w260:i32)
                    n266 = Replace Array Subset(array=w262, new element=w261, index (col)=w260) -> (w263:dbl[][])  [unwired: 1 in]
                    n267 = property on="强度图" class="IntGraph (严格)"("Value"=w263) -> ()  [unwired: 2 in, 2 out]
                    n268 = Equal?(x=w260, y=w274) -> (x = y?=w280:bool)
                    n269 = Increment(x=w260) -> ()  [unwired: 1 out]
                    n270 = flat-sequence {
                      tunnel: w256 -> [w286]
                      tunnel: [w286] -> w255
                      frame #0 {
                        n271 = local read "毫秒计时值"() -> (w281:u32)
                        n272 = Tick Count (ms)() -> (millisecond timer value=w285:u32)
                        n273 = Subtract(x=w285, y=w281) -> (x-y=w282:u32)
                        n274 = Multiply(x=w282, y=0.001) -> (x*y=→"已用时（s）":dbl)
                      }
                    }
                    n275 = property on="细分设置" class="DigNum (严格)"() -> ("Value"=w266:dbl)  [unwired: 2 in, 2 out]
                    n276 = property on="等待时间" class="DigNum (严格)"() -> ("Value"=w267:u32)  [unwired: 2 in, 2 out]
                    n277 = case shown="假" w280 {
                      tunnel: w255 -> [w364 w396]
                      tunnel: [w362 w397] -> w278
                      tunnel: w267 -> [w360 w394]
                      tunnel: w266 -> [w359 w393]
                      frame False {
                        n278 = flat-sequence {
                          tunnel: w364 -> [w368]
                          tunnel: [w368] -> w363
                          tunnel: [w366] -> w361
                          tunnel: w360 -> [w367]
                          tunnel: w359 -> [w366]
                          frame #0 {
                            n279 = call "X,Y,Z轴坐标查询.vi"("细分设置"=w366, "查询坐标轴"="Y", "串口通信端口"=w368) -> ("坐标(mm)"=w369:dbl)
                            n280 = property on="Y:" class="DigNum (严格)"() -> ("Value"=w365:dbl)  [unwired: 2 in, 2 out]
                            n281 = Add(x=w369, y=w365) -> (x+y=w371:dbl)
                            "x+y 2" <- w371
                            n282 = Multiply(x=w371, y=200.0) -> (x*y=w375:dbl)
                            n283 = Multiply(x=w375, y=8.0 ("细分设置")) -> (x*y=w380:dbl)
                            n284 = Number To Fractional String(number=w380, precision (6)=i16 0 ("精度(6)")) -> (F-format string=w378:string)  [unwired: 2 out]
                            n285 = Concatenate Strings("Y=" ("字符串"), w378, "/" ("字符串")) -> (w373:string)
                            n286 = call "步进电机命令输入与输出.vi"("输入字符串"=w373, "串口通信端口"=w368) -> ()  [unwired: 1 out]
                            n287 = Wait (ms)(milliseconds to wait=w367) -> ()  [unwired: 1 out]
                          }
                        }
                        n288 = while {
                          shift-right: [w382] -> w362
                          shift-left: w363 -> [w382]
                          shift-right: [w381] -> _
                          shift-left: w361 -> [w381]
                          stop <- w388 stop-if-true
                          n289 = call "X,Y,Z轴坐标查询.vi"("细分设置"=w381, "查询坐标轴"="Y", "串口通信端口"=w382) -> ("坐标(mm)"=w386:dbl)
                          n290 = local read "x+y 2"() -> (w389:dbl)
                          n291 = property on="电机急停" class="Bool (严格)"() -> ("Value"=w385:bool)  [unwired: 2 in, 2 out]
                          n292 = property on="Y(mm)" class="DigNum (严格)"("Value"=w386) -> ()  [unwired: 2 in, 2 out]
                          n293 = case shown="真" w385 {
                            tunnel: w382 -> [_ w391]
                            frame False {
                            }
                            frame True {
                              n294 = call "步进电机命令输入与输出.vi"("输入字符串"="S0/", "串口通信端口"=w391) -> ()  [unwired: 1 out]
                            }
                          }
                          n295 = Subtract(x=w389, y=w386) -> (x-y=w384:dbl)
                          n296 = Absolute Value(x=w384) -> (abs(x)=w383:dbl)
                          n297 = local read "精度"() -> (w387:dbl)
                          n298 = Less?(x=w383, y=w387) -> (x < y?=w388:bool)
                        }
                      }
                      frame True {
                        n299 = flat-sequence {
                          tunnel: [w401] -> _
                          tunnel: [w401] -> w398
                          tunnel: w396 -> [w401]
                          tunnel: [w399] -> w395
                          tunnel: w394 -> [w400]
                          tunnel: w393 -> [w399]
                          frame #0 {
                            n300 = Multiply(x=0.0, y=200.0) -> (x*y=w405:dbl)
                            n301 = Multiply(x=w405, y=w399) -> (x*y=w410:dbl)
                            n302 = Number To Fractional String(number=w410, precision (6)=i16 0 ("精度(6)")) -> (F-format string=w408:string)  [unwired: 2 out]
                            n303 = Concatenate Strings("Y=" ("字符串"), w408, "/" ("字符串")) -> (w403:string)
                            n304 = call "步进电机命令输入与输出.vi"("输入字符串"=w403, "串口通信端口"=w401) -> ()  [unwired: 1 out]
                            n305 = Wait (ms)(milliseconds to wait=w400) -> ()  [unwired: 1 out]
                          }
                        }
                        n306 = while {
                          shift-right: [w412] -> w397
                          shift-left: w398 -> [w412]
                          shift-right: [w411] -> _
                          shift-left: w395 -> [w411]
                          stop <- w418 stop-if-true
                          n307 = property on="电机急停" class="Bool (严格)"() -> ("Value"=w419:bool)  [unwired: 2 in, 2 out]
                          n308 = call "X,Y,Z轴坐标查询.vi"("细分设置"=w411, "查询坐标轴"="Y", "串口通信端口"=w412) -> ("坐标(mm)"=w420:dbl)
                          n309 = case shown="真" w419 {
                            tunnel: w412 -> [_ w423]
                            frame False {
                            }
                            frame True {
                              n310 = call "步进电机命令输入与输出.vi"("输入字符串"="S0/", "串口通信端口"=w423) -> ()  [unwired: 1 out]
                            }
                          }
                          n311 = Multiply(x=w420, y=1.0 ("x")) -> (x*y=w416:dbl)
                          n312 = Subtract(x=w416, y=0.0 ("x")) -> (x-y=w414:dbl)
                          n313 = local read "精度"() -> (w417:dbl)
                          n314 = Absolute Value(x=w414) -> (abs(x)=w413:dbl)
                          n315 = property on="Y(mm)" class="DigNum (严格)"("Value"=w416) -> ()  [unwired: 2 in, 2 out]
                          n316 = Less?(x=w413, y=w417) -> (x < y?=w418:bool)
                        }
                      }
                    }
                    "Y序" <- w279
                  }
                  n317 = property on="已用时（s）" class="DigNum (严格)"("Visible"=TRUE ("可见")) -> ()  [unwired: 2 in, 2 out]
                  n318 = flat-sequence {
                    tunnel: [w204] -> w187
                    tunnel: ["文件保存"] -> w185
                    tunnel: w185 -> [w209]
                    tunnel: [w208] -> w184
                    frame #0 {
                      n319 = Build Path(base path="文件保存", name or relative path="频域谱" ("名称或相对路径")) -> (appended path=w207:path)
                      n320 = Create Folder(path (use dialog)=w207) -> (created path=w204:path)  [unwired: 2 in, 2 out]
                    }
                    frame #1 {
                      n321 = Build Path(base path=w209, name or relative path="时域谱" ("名称或相对路径")) -> (appended path=w210:path)
                      n322 = Create Folder(path (use dialog)=w210) -> (created path=w208:path)  [unwired: 2 in, 2 out]
                    }
                  }
                  n323 = flat-sequence {
                    tunnel: w199 -> [w214]
                    tunnel: [w212] -> _
                    tunnel: [w212] -> w181
                    tunnel: [w214] -> w180
                    tunnel: w179 -> [w212]
                    tunnel: [w215] -> w198
                    tunnel: w181 -> [w215]
                    tunnel: w180 -> [w218]
                    frame #0 {
                      n324 = property on="水平进度条" class="Slide (严格)"("Value"=u8 100 ("水平进度条")) -> ()  [unwired: 2 in, 2 out]
                    }
                    frame #1 {
                      n325 = local read "毫秒计时值"() -> (w217:u32)
                      n326 = Tick Count (ms)() -> (millisecond timer value=w222:u32)
                      n327 = Transpose 2D Array(2D array=w218) -> (transposed array=w219:dbl[][])
                      n328 = Subtract(x=w222, y=w217) -> (x-y=w220:u32)
                      n329 = property on="强度图" class="IntGraph (严格)"("Value"=w219) -> ()  [unwired: 2 in, 2 out]
                      n330 = Multiply(x=w220, y=0.001) -> (x*y=w216:dbl)
                      n331 = property on="已用时（s）" class="DigNum (严格)"("Value"=w216) -> ()  [unwired: 2 in, 2 out]
                      "数组" <- w218
                    }
                  }
                }
                event "逐行扫描": Value Change {
                  n332 = event-data() -> ()  [unwired: 1 in, 6 out]
                  n333 = flat-sequence {
                    tunnel: [w608] -> w521
                    tunnel: [w607] -> w518
                    tunnel: w521 -> [w612]
                    tunnel: [w611] -> w520
                    frame #0 {
                      n334 = local read "文件保存"() -> (w608:path)
                      n335 = Build Path(base path=w608, name or relative path="频域谱" ("名称或相对路径")) -> (appended path=w610:path)
                      n336 = Create Folder(path (use dialog)=w610) -> (created path=w607:path)  [unwired: 2 in, 2 out]
                    }
                    frame #1 {
                      n337 = Build Path(base path=w612, name or relative path="时域谱" ("名称或相对路径")) -> (appended path=w613:path)
                      n338 = Create Folder(path (use dialog)=w613) -> (created path=w611:path)  [unwired: 2 in, 2 out]
                    }
                  }
                  n339 = flat-sequence {
                    tunnel: [w565] -> w516
                    tunnel: w517 -> [w565]
                    frame #0 {
                      # "如果强度图那里出了错，就把这里的行列互换"
                      n340 = property on="Y起点" class="DigNum (严格)"() -> ("Value"=w568:dbl)  [unwired: 2 in, 2 out]
                      n341 = property on="细分设置" class="DigNum (严格)"() -> ("Value"=w566:dbl)  [unwired: 2 in, 2 out]
                      n342 = local read "Xloop"() -> (w572:dbl)
                      n343 = local read "Yloop"() -> (w571:dbl)
                      n344 = Multiply(x=w568, y=200.0) -> (x*y=w576:dbl)
                      n345 = Tick Count (ms)() -> (millisecond timer value=w569:u32)
                      n346 = Multiply(x=w576, y=w566) -> (x*y=w581:dbl)
                      n347 = Initialize Array(0.0 ("元素"), w572, w571) -> (w567:dbl[][])
                      n348 = Number To Fractional String(number=w581, precision (6)=i16 0 ("精度(6)")) -> (F-format string=w579:string)  [unwired: 2 out]
                      n349 = property on="毫秒计时值" class="DigNum (严格)"("Value"=w569) -> ()  [unwired: 2 in, 2 out]
                      n350 = property on="强度图" class="IntGraph (严格)"("Value"=w567) -> ()  [unwired: 2 in, 2 out]
                      n351 = Concatenate Strings("Y=" ("字符串"), w579, "/" ("字符串")) -> (w574:string)
                      n352 = call "步进电机命令输入与输出.vi"("输入字符串"=w574, "串口通信端口"=w565) -> ()  [unwired: 1 out]
                      n353 = property on="等待时间" class="DigNum (严格)"() -> ("Value"=w570:u32)  [unwired: 2 in, 2 out]
                      n354 = property on="已用时（s）" class="DigNum (严格)"("Value"=0.0 ("已用时（s）")) -> ()  [unwired: 2 in, 2 out]
                      n355 = Wait (ms)(milliseconds to wait=w570) -> ()  [unwired: 1 out]
                    }
                  }
                  n356 = property on="水平进度条" class="Slide (严格)"("Visible"=TRUE ("可见")) -> ()  [unwired: 2 in, 2 out]
                  n357 = property on="单行？" class="RadioBtnsControl (严格)"("Visible"=FALSE ("可见")) -> ()  [unwired: 2 in, 2 out]
                  n358 = flat-sequence {
                    tunnel: [w560] -> w515
                    frame #0 {
                      n359 = property on="X终点" class="DigNum (严格)"() -> ("Value"=w549:dbl)  [unwired: 2 in, 2 out]
                      n360 = property on="X起点" class="DigNum (严格)"() -> ("Value"=w548:dbl)  [unwired: 2 in, 2 out]
                      n361 = Subtract(x=w549, y=w548) -> (x-y=w553:dbl)
                      n362 = local read "X:"() -> (w552:dbl)
                      n363 = property on="X扫描范围" class="DigNum (严格)"("Value"=w553) -> ()  [unwired: 2 in, 2 out]
                      n364 = Divide(x=w553, y=w552) -> (x/y=w551:dbl)
                      n365 = Increment(x=w551) -> (x+1=w550:dbl)
                      n366 = property on="Xloop" class="DigNum (严格)"("Value"=w550) -> ()  [unwired: 2 in, 2 out]
                    }
                    frame #1 {
                      n367 = property on="Y终点" class="DigNum (严格)"() -> ("Value"=w555:dbl)  [unwired: 2 in, 2 out]
                      n368 = property on="Y起点" class="DigNum (严格)"() -> ("Value"=w554:dbl)  [unwired: 2 in, 2 out]
                      n369 = Subtract(x=w555, y=w554) -> (x-y=w558:dbl)
                      n370 = local read "Y:"() -> (w557:dbl)
                      n371 = property on="Y扫描范围" class="DigNum (严格)"("Value"=w558) -> ()  [unwired: 2 in, 2 out]
                      n372 = Divide(x=w558, y=w557) -> (x/y=w559:dbl)
                      n373 = Increment(x=w559) -> (x+1=w556:dbl)
                      n374 = property on="Yloop" class="DigNum (严格)"("Value"=w556) -> ()  [unwired: 2 in, 2 out]
                    }
                    frame #2 {
                      n375 = property on="Xloop" class="DigNum (严格)"() -> ("Value"=w563:dbl)  [unwired: 2 in, 2 out]
                      n376 = property on="Yloop" class="DigNum (严格)"() -> ("Value"=w560:dbl)  [unwired: 2 in, 2 out]
                      n377 = Initialize Array(0.0 ("元素"), w563, w560) -> (w562:dbl[][])
                      n378 = property on="强度图" class="IntGraph (严格)"("Value"=w562) -> ()  [unwired: 2 in, 2 out]
                    }
                  }
                  n379 = while {
                    shift-right: [w583] -> w505
                    shift-left: w516 -> [w583]
                    stop <- w588 stop-if-true
                    n380 = call "X,Y,Z轴坐标查询.vi"("细分设置"=8.0, "查询坐标轴"="Y", "串口通信端口"=w583) -> ("坐标(mm)"=w590:dbl)
                    n381 = property on="Y起点" class="DigNum (严格)"() -> ("Value"=w582:dbl)  [unwired: 2 in, 2 out]
                    n382 = property on="电机急停" class="Bool (严格)"() -> ("Value"=w589:bool)  [unwired: 2 in, 2 out]
                    n383 = Multiply(x=w590, y=1.0 ("x")) -> (x*y=w586:dbl)
                    n384 = Subtract(x=w582, y=w586) -> (x-y=w585:dbl)
                    n385 = case shown="真" w589 {
                      tunnel: w583 -> [_ w594]
                      frame False {
                      }
                      frame True {
                        n386 = call "步进电机命令输入与输出.vi"("输入字符串"="S0/", "串口通信端口"=w594) -> ()  [unwired: 1 out]
                      }
                    }
                    n387 = Absolute Value(x=w585) -> (abs(x)=w584:dbl)
                    n388 = local read "精度"() -> (w587:dbl)
                    n389 = property on="Y(mm)" class="DigNum (严格)"("Value"=w586) -> ()  [unwired: 2 in, 2 out]
                    n390 = Less?(x=w584, y=w587) -> (x < y?=w588:bool)
                  }
                  n391 = flat-sequence {
                    tunnel: w505 -> [w525]
                    tunnel: [w525] -> w507
                    tunnel: [w522] -> w506
                    frame #0 {
                      n392 = property on="细分设置" class="DigNum (严格)"() -> ("Value"=w522:dbl)  [unwired: 2 in, 2 out]
                      n393 = Multiply(x=0.0, y=50.0) -> (x*y=w528:dbl)
                      n394 = Multiply(x=w528, y=w522) -> (x*y=w533:dbl)
                      n395 = Number To Fractional String(number=w533, precision (6)=i16 0 ("精度(6)")) -> (F-format string=w531:string)  [unwired: 2 out]
                      n396 = Concatenate Strings("X=" ("字符串"), w531, "/" ("字符串")) -> (w526:string)
                      n397 = call "步进电机命令输入与输出.vi"("输入字符串"=w526, "串口通信端口"=w525) -> ()  [unwired: 1 out]
                      n398 = property on="等待时间" class="DigNum (严格)"() -> ("Value"=w523:u32)  [unwired: 2 in, 2 out]
                      n399 = Wait (ms)(milliseconds to wait=w523) -> ()  [unwired: 1 out]
                    }
                  }
                  n400 = while {
                    shift-right: [w535] -> w504
                    shift-left: w507 -> [w535]
                    shift-right: [w534] -> _
                    shift-left: w506 -> [w534]
                    stop <- w541 stop-if-true
                    n401 = property on="电机急停" class="Bool (严格)"() -> ("Value"=w542:bool)  [unwired: 2 in, 2 out]
                    n402 = call "X,Y,Z轴坐标查询.vi"("细分设置"=w534, "查询坐标轴"="X", "串口通信端口"=w535) -> ("坐标(mm)"=w543:dbl)
                    n403 = case shown="真" w542 {
                      tunnel: w535 -> [_ w546]
                      frame False {
                      }
                      frame True {
                        n404 = call "步进电机命令输入与输出.vi"("输入字符串"="S0/", "串口通信端口"=w546) -> ()  [unwired: 1 out]
                      }
                    }
                    n405 = Multiply(x=w543, y=4.0 ("x")) -> (x*y=w539:dbl)
                    n406 = Subtract(x=0.0, y=w539) -> (x-y=w538:dbl)
                    n407 = Absolute Value(x=w538) -> (abs(x)=w537:dbl)
                    n408 = local read "精度"() -> (w540:dbl)
                    n409 = property on="X（mm）" class="DigNum (严格)"("Value"=w539) -> ()  [unwired: 2 in, 2 out]
                    n410 = Less?(x=w537, y=w540) -> (x < y?=w541:bool)
                  }
                  n411 = for {
                    N: w515 -> [_]
                    shift-right: [w630] -> _
                    shift-left: w518 -> [w630]
                    shift-right: [w629] -> _
                    shift-left: w520 -> [w629]
                    tunnel: [w628] -> w514 mode=indexing
                    shift-right: [w621] -> w513
                    shift-left: w504 -> [w623]
                    i -> [w616]
                    # "实时成像出问题调这里"
                    n412 = local read "Yloop"() -> (w618:dbl)
                    n413 = property on="Y序" class="DigNum (严格)"("Value"=w616) -> ()  [unwired: 2 in, 2 out]
                    n414 = Multiply(x=w618, y=0.01) -> (x*y=w617:dbl)
                    n415 = Divide(x=w616, y=w617) -> (x/y=w619:dbl)
                    n416 = property on="水平进度条" class="Slide (严格)"("Value"=w619) -> ()  [unwired: 2 in, 2 out]
                    n417 = case shown="\"双行\"" "单行？" {
                      tunnel: w630 -> [w641 w716]
                      tunnel: w629 -> [w640 w717]
                      tunnel: [w639 w713] -> w628
                      tunnel: [w635 w711] -> w626
                      tunnel: w623 -> [w634 w715]
                      frame "单行", Default {
                        n418 = flat-sequence {
                          tunnel: [w675] -> w644
                          tunnel: [w673] -> w643
                          tunnel: [w676] -> w639
                          tunnel: [w674] -> w642
                          tunnel: w634 -> [w672]
                          tunnel: [w706] -> w636
                          tunnel: w640 -> [w690]
                          tunnel: w641 -> [w689]
                          tunnel: w644 -> [w702]
                          tunnel: w643 -> [w706]
                          tunnel: w642 -> [w694]
                          frame #0 {
                            n419 = local read "精度"() -> (w684:dbl)
                            n420 = property on="细分设置" class="DigNum (严格)"() -> ("Value"=w683:dbl)  [unwired: 2 in, 2 out]
                            n421 = property on="X终点" class="DigNum (严格)"() -> ("Value"=w687:dbl)  [unwired: 2 in, 2 out]
                            n422 = property on="X起点" class="DigNum (严格)"() -> ("Value"=w671:dbl)  [unwired: 2 in, 2 out]
                            n423 = local read "待读取数据长度"() -> (w679:i32)
                            n424 = local read "M_Length"() -> (w681:i32)
                            n425 = property on="hDevice" class="DigNum (严格)"() -> ("Value"=w680:i32)  [unwired: 2 in, 2 out]
                            n426 = property on="N_Length" class="DigNum (严格)"() -> ("Value"=w682:i32)  [unwired: 2 in, 2 out]
                            n427 = property on="等待时间" class="DigNum (严格)"() -> ("Value"=w685:u32)  [unwired: 2 in, 2 out]
                            n428 = property on="电机急停" class="Bool (严格)"() -> ("Value"=w686:bool)  [unwired: 2 in, 2 out]
                            n429 = call "X轴连续扫描（1.0）.vi"("VISA I"=w672, "X0"=w671, "X"=w687, "精度"=w684, "细分设置"=w683, "等待时间(ms)"=w685, "pulDDR2Length"=w679, "电机急停"=w686, "hDevice"=w680, "M-length"=w681, "N-length"=w682) -> ("VISA O"=w673:refnum<visa-resource-name>, "hDevice out"=w678:i32, "X"=w677:dbl, "强度图行"=w676:dbl[], "时域谱页"=w675:dbl[][], "幅频谱页"=w674:dbl[][])  [unwired: 3 in]
                            n430 = property on="hDevice 2" class="DigNum (严格)"("Value"=w678) -> ()  [unwired: 2 in, 2 out]
                            n431 = property on="X（mm）" class="DigNum (严格)"("Value"=w677) -> ()  [unwired: 2 in, 2 out]
                          }
                          frame #1 {
                            n432 = property on="Y序" class="DigNum (严格)"() -> ("Value"=w688:i32)  [unwired: 2 in, 2 out]
                            n433 = Increment(x=w688) -> (x+1=w691:i32)
                            n434 = Number To Decimal String(number=w691) -> (decimal integer string=w700:string)  [unwired: 1 in]
                            n435 = Number To Decimal String(number=w691) -> (decimal integer string=w699:string)  [unwired: 1 in]
                            n436 = Concatenate Strings("T" ("字符串"), w700, ".txt" ("字符串")) -> (w703:string)
                            n437 = Concatenate Strings("F" ("字符串"), w699, ".txt" ("字符串")) -> (w697:string)
                            n438 = Build Path(base path=w690, name or relative path=w703) -> (appended path=w705:path)
                            n439 = call-poly <vilib>:"Write Delimited Spreadsheet.vi"("file path (dialog if empty)"=w705, "2D data"=w702, "transpose? (no:F)"=FALSE) -> ()  [unwired: 11 in, 2 out]
                            n440 = Build Path(base path=w689, name or relative path=w697) -> (appended path=w695:path)
                            n441 = call-poly <vilib>:"Write Delimited Spreadsheet.vi"("file path (dialog if empty)"=w695, "2D data"=w694, "transpose? (no:F)"=FALSE) -> ()  [unwired: 11 in, 2 out]
                          }
                        }
                        n442 = flat-sequence {
                          tunnel: w636 -> [w648]
                          tunnel: [w648] -> w637
                          tunnel: [w647] -> w638
                          frame #0 {
                            n443 = property on="细分设置" class="DigNum (严格)"() -> ("Value"=w647:dbl)  [unwired: 2 in, 2 out]
                            n444 = Multiply(x=0.0, y=50.0) -> (x*y=w651:dbl)
                            n445 = Multiply(x=w651, y=w647) -> (x*y=w656:dbl)
                            n446 = local read "等待时间"() -> (w646:u32)
                            n447 = Number To Fractional String(number=w656, precision (6)=i16 0 ("精度(6)")) -> (F-format string=w654:string)  [unwired: 2 out]
                            n448 = Concatenate Strings("X=" ("字符串"), w654, "/" ("字符串")) -> (w649:string)
                            n449 = Wait (ms)(milliseconds to wait=w646) -> ()  [unwired: 1 out]
                            n450 = call "步进电机命令输入与输出.vi"("输入字符串"=w649, "串口通信端口"=w648) -> ()  [unwired: 1 out]
                          }
                        }
                        n451 = while {
                          shift-right: [w660] -> w635
                          shift-left: w637 -> [w660]
                          shift-right: [w658] -> _
                          shift-left: w638 -> [w658]
                          stop <- w664 stop-if-true
                          n452 = property on="电机急停" class="Bool (严格)"() -> ("Value"=w665:bool)  [unwired: 2 in, 2 out]
                          n453 = case shown="真" w665 {
                            tunnel: w660 -> [_ w669]
                            frame False {
                            }
                            frame True {
                              n454 = call "步进电机命令输入与输出.vi"("输入字符串"="S0/", "串口通信端口"=w669) -> ()  [unwired: 1 out]
                            }
                          }
                          n455 = call "X,Y,Z轴坐标查询.vi"("细分设置"=w658, "查询坐标轴"="X", "串口通信端口"=w660) -> ("坐标(mm)"=w666:dbl)
                          n456 = Multiply(x=w666, y=4.0 ("x")) -> (x*y=w662:dbl)
                          n457 = Subtract(x=0.0, y=w662) -> (x-y=w661:dbl)
                          n458 = local read "精度"() -> (w663:dbl)
                          n459 = Absolute Value(x=w661) -> (abs(x)=w659:dbl)
                          n460 = property on="X（mm）" class="DigNum (严格)"("Value"=w662) -> ()  [unwired: 2 in, 2 out]
                          n461 = Less?(x=w659, y=w663) -> (x < y?=w664:bool)
                        }
                      }
                      frame "双行" {
                        n462 = flat-sequence {
                          tunnel: [w758] -> w720
                          tunnel: [w756] -> w719
                          tunnel: [w759] -> w713
                          tunnel: [w757] -> w718
                          tunnel: w715 -> [w755]
                          tunnel: [w752] -> w714
                          tunnel: [w812] -> w712
                          tunnel: w717 -> [w796]
                          tunnel: w716 -> [w795]
                          tunnel: w720 -> [w808]
                          tunnel: w719 -> [w812]
                          tunnel: w718 -> [w800]
                          tunnel: w714 -> [w794]
                          tunnel: [w794] -> w707
                          frame #0 {
                            n463 = property on="Y序" class="DigNum (严格)"() -> ("Value"=w752:i32)  [unwired: 2 in, 2 out]
                            n464 = Power Of X(1:-1.0 ("x"), 2:w752) -> (0:w753:dbl)
                            n465 = case shown="-1" w753 {
                              tunnel: [w761 w782] -> w759
                              tunnel: [w764 w781] -> w758
                              tunnel: [w763 w780] -> w757
                              tunnel: [w762 w779] -> w756
                              tunnel: w755 -> [w760 w778]
                              frame -1 {
                                n466 = local read "精度"() -> (w773:dbl)
                                n467 = property on="细分设置" class="DigNum (严格)"() -> ("Value"=w772:dbl)  [unwired: 2 in, 2 out]
                                n468 = property on="X终点" class="DigNum (严格)"() -> ("Value"=w776:dbl)  [unwired: 2 in, 2 out]
                                n469 = property on="X起点" class="DigNum (严格)"() -> ("Value"=w765:dbl)  [unwired: 2 in, 2 out]
                                n470 = local read "量程选择"() -> (w768:i32)
                                n471 = local read "M_Length"() -> (w770:i32)
                                n472 = property on="hDevice" class="DigNum (严格)"() -> ("Value"=w769:i32)  [unwired: 2 in, 2 out]
                                n473 = property on="N_Length" class="DigNum (严格)"() -> ("Value"=w771:i32)  [unwired: 2 in, 2 out]
                                n474 = property on="等待时间" class="DigNum (严格)"() -> ("Value"=w774:u32)  [unwired: 2 in, 2 out]
                                n475 = property on="电机急停" class="Bool (严格)"() -> ("Value"=w775:bool)  [unwired: 2 in, 2 out]
                                n476 = call "X轴回程连续扫描（1.0）.vi"("VISA I"=w760, "X0"=w765, "X"=w776, "精度"=w773, "细分设置"=w772, "等待时间(ms)"=w774, "pulDDR2Length"=w768, "电机急停"=w775, "hDevice"=w769, "M-length"=w770, "N-length"=w771) -> ("VISA O"=w762:refnum<visa-resource-name>, "hDevice out"=w767:i32, "X"=w766:dbl, "强度图行"=w761:dbl[], "时域谱页"=w764:dbl[][], "幅频谱页"=w763:dbl[][])  [unwired: 3 in]
                                n477 = property on="X（mm）" class="DigNum (严格)"("Value"=w766) -> ()  [unwired: 2 in, 2 out]
                                n478 = property on="hDevice 2" class="DigNum (严格)"("Value"=w767) -> ()  [unwired: 2 in, 2 out]
                              }
                              frame 1, Default {
                                n479 = local read "精度"() -> (w790:dbl)
                                n480 = property on="细分设置" class="DigNum (严格)"() -> ("Value"=w789:dbl)  [unwired: 2 in, 2 out]
                                n481 = property on="X终点" class="DigNum (严格)"() -> ("Value"=w793:dbl)  [unwired: 2 in, 2 out]
                                n482 = property on="X起点" class="DigNum (严格)"() -> ("Value"=w777:dbl)  [unwired: 2 in, 2 out]
                                n483 = local read "量程选择"() -> (w785:i32)
                                n484 = local read "M_Length"() -> (w787:i32)
                                n485 = property on="hDevice" class="DigNum (严格)"() -> ("Value"=w786:i32)  [unwired: 2 in, 2 out]
                                n486 = property on="N_Length" class="DigNum (严格)"() -> ("Value"=w788:i32)  [unwired: 2 in, 2 out]
                                n487 = property on="等待时间" class="DigNum (严格)"() -> ("Value"=w791:u32)  [unwired: 2 in, 2 out]
                                n488 = property on="电机急停" class="Bool (严格)"() -> ("Value"=w792:bool)  [unwired: 2 in, 2 out]
                                n489 = call "X轴连续扫描（1.0）.vi"("VISA I"=w778, "X0"=w777, "X"=w793, "精度"=w790, "细分设置"=w789, "等待时间(ms)"=w791, "pulDDR2Length"=w785, "电机急停"=w792, "hDevice"=w786, "M-length"=w787, "N-length"=w788) -> ("VISA O"=w779:refnum<visa-resource-name>, "hDevice out"=w784:i32, "X"=w783:dbl, "强度图行"=w782:dbl[], "时域谱页"=w781:dbl[][], "幅频谱页"=w780:dbl[][])  [unwired: 3 in]
                                n490 = property on="hDevice 2" class="DigNum (严格)"("Value"=w784) -> ()  [unwired: 2 in, 2 out]
                                n491 = property on="X（mm）" class="DigNum (严格)"("Value"=w783) -> ()  [unwired: 2 in, 2 out]
                              }
                            }
                          }
                          frame #1 {
                            n492 = Increment(x=w794) -> (x+1=w797:i32)
                            n493 = Number To Decimal String(number=w797) -> (decimal integer string=w806:string)  [unwired: 1 in]
                            n494 = Number To Decimal String(number=w797) -> (decimal integer string=w805:string)  [unwired: 1 in]
                            n495 = Concatenate Strings("T" ("字符串"), w806, ".txt" ("字符串")) -> (w809:string)
                            n496 = Concatenate Strings("F" ("字符串"), w805, ".txt" ("字符串")) -> (w803:string)
                            n497 = Build Path(base path=w796, name or relative path=w809) -> (appended path=w811:path)
                            n498 = call-poly <vilib>:"Write Delimited Spreadsheet.vi"("file path (dialog if empty)"=w811, "2D data"=w808, "transpose? (no:F)"=FALSE) -> ()  [unwired: 11 in, 2 out]
                            n499 = Build Path(base path=w795, name or relative path=w803) -> (appended path=w801:path)
                            n500 = call-poly <vilib>:"Write Delimited Spreadsheet.vi"("file path (dialog if empty)"=w801, "2D data"=w800, "transpose? (no:F)"=FALSE) -> ()  [unwired: 11 in, 2 out]
                          }
                        }
                        n501 = property on="Yloop" class="DigNum (严格)"() -> ("Value"=w710:dbl)  [unwired: 2 in, 2 out]
                        n502 = Decrement(x=w710) -> (x-1=w709:dbl)
                        n503 = Equal?(x=w707, y=w709) -> (x = y?=w708:bool)
                        n504 = case shown="假" w708 {
                          tunnel: w712 -> [w721 w722]
                          tunnel: [w721 w723] -> w711
                          frame False {
                          }
                          frame True {
                            n505 = flat-sequence {
                              tunnel: w722 -> [w729]
                              tunnel: [w729] -> w724
                              tunnel: [w728] -> w725
                              frame #0 {
                                n506 = property on="细分设置" class="DigNum (严格)"() -> ("Value"=w728:dbl)  [unwired: 2 in, 2 out]
                                n507 = Multiply(x=0.0, y=50.0) -> (x*y=w732:dbl)
                                n508 = Multiply(x=w732, y=w728) -> (x*y=w737:dbl)
                                n509 = local read "等待时间"() -> (w727:u32)
                                n510 = Number To Fractional String(number=w737, precision (6)=i16 0 ("精度(6)")) -> (F-format string=w735:string)  [unwired: 2 out]
                                n511 = Concatenate Strings("X=" ("字符串"), w735, "/" ("字符串")) -> (w730:string)
                                n512 = Wait (ms)(milliseconds to wait=w727) -> ()  [unwired: 1 out]
                                n513 = call "步进电机命令输入与输出.vi"("输入字符串"=w730, "串口通信端口"=w729) -> ()  [unwired: 1 out]
                              }
                            }
                            n514 = while {
                              shift-right: [w741] -> w723
                              shift-left: w724 -> [w741]
                              shift-right: [w739] -> _
                              shift-left: w725 -> [w739]
                              stop <- w745 stop-if-true
                              n515 = property on="电机急停" class="Bool (严格)"() -> ("Value"=w746:bool)  [unwired: 2 in, 2 out]
                              n516 = case shown="真" w746 {
                                tunnel: w741 -> [_ w750]
                                frame False {
                                }
                                frame True {
                                n517 = call "步进电机命令输入与输出.vi"("输入字符串"="S0/", "串口通信端口"=w750) -> ()  [unwired: 1 out]
                                }
                              }
                              n518 = call "X,Y,Z轴坐标查询.vi"("细分设置"=w739, "查询坐标轴"="X", "串口通信端口"=w741) -> ("坐标(mm)"=w747:dbl)
                              n519 = Multiply(x=w747, y=4.0 ("x")) -> (x*y=w743:dbl)
                              n520 = Subtract(x=0.0, y=w743) -> (x-y=w742:dbl)
                              n521 = local read "精度"() -> (w744:dbl)
                              n522 = Absolute Value(x=w742) -> (abs(x)=w740:dbl)
                              n523 = property on="X（mm）" class="DigNum (严格)"("Value"=w743) -> ()  [unwired: 2 in, 2 out]
                              n524 = Less?(x=w740, y=w744) -> (x < y?=w745:bool)
                            }
                          }
                        }
                      }
                    }
                    n525 = property on="强度图" class="IntGraph (严格)"() -> ("Value"=w633:dbl[][])  [unwired: 2 in, 2 out]
                    n526 = property on="Yloop" class="DigNum (严格)"() -> ("Value"=w624:dbl)  [unwired: 2 in, 2 out]
                    n527 = property on="Y序" class="DigNum (严格)"() -> ("Value"=w627:i32)  [unwired: 2 in, 2 out]
                    n528 = Replace Array Subset(array=w633, new element=w628, index (col)=w627) -> (w632:dbl[][])  [unwired: 1 in]
                    n529 = property on="强度图" class="IntGraph (严格)"("Value"=w632) -> ()  [unwired: 2 in, 2 out]
                    n530 = Decrement(x=w624) -> (x-1=w625:dbl)
                    n531 = Equal?(x=w627, y=w625) -> (x = y?=w631:bool)
                    n532 = case shown="真" w631 {
                      tunnel: w626 -> [w822 w852]
                      tunnel: [w820 w853] -> w622
                      frame False {
                        n533 = flat-sequence {
                          tunnel: w822 -> [w826]
                          tunnel: [w826] -> w821
                          tunnel: [w823] -> w819
                          frame #0 {
                            n534 = property on="细分设置" class="DigNum (严格)"() -> ("Value"=w823:dbl)  [unwired: 2 in, 2 out]
                            n535 = call "X,Y,Z轴坐标查询.vi"("细分设置"=w823, "查询坐标轴"="Y", "串口通信端口"=w826) -> ("坐标(mm)"=w827:dbl)
                            n536 = property on="Y:" class="DigNum (严格)"() -> ("Value"=w825:dbl)  [unwired: 2 in, 2 out]
                            n537 = Add(x=w827, y=w825) -> (x+y=w829:dbl)
                            "x+y 3" <- w829
                            n538 = Multiply(x=w829, y=200.0) -> (x*y=w833:dbl)
                            n539 = Multiply(x=w833, y=8.0 ("细分设置")) -> (x*y=w838:dbl)
                            n540 = Number To Fractional String(number=w838, precision (6)=i16 0 ("精度(6)")) -> (F-format string=w836:string)  [unwired: 2 out]
                            n541 = Concatenate Strings("Y=" ("字符串"), w836, "/" ("字符串")) -> (w831:string)
                            n542 = call "步进电机命令输入与输出.vi"("输入字符串"=w831, "串口通信端口"=w826) -> ()  [unwired: 1 out]
                            n543 = property on="等待时间" class="DigNum (严格)"() -> ("Value"=w824:u32)  [unwired: 2 in, 2 out]
                            n544 = Wait (ms)(milliseconds to wait=w824) -> ()  [unwired: 1 out]
                          }
                        }
                        n545 = while {
                          shift-right: [w841] -> w820
                          shift-left: w821 -> [w841]
                          shift-right: [w840] -> _
                          shift-left: w819 -> [w840]
                          stop <- w847 stop-if-true
                          n546 = call "X,Y,Z轴坐标查询.vi"("细分设置"=w840, "查询坐标轴"="Y", "串口通信端口"=w841) -> ("坐标(mm)"=w845:dbl)
                          n547 = property on="x+y 3" class="DigNum (严格)"() -> ("Value"=w839:dbl)  [unwired: 2 in, 2 out]
                          n548 = property on="电机急停" class="Bool (严格)"() -> ("Value"=w844:bool)  [unwired: 2 in, 2 out]
                          n549 = property on="Y(mm)" class="DigNum (严格)"("Value"=w845) -> ()  [unwired: 2 in, 2 out]
                          n550 = case shown="真" w844 {
                            tunnel: w841 -> [_ w849]
                            frame False {
                            }
                            frame True {
                              n551 = call "步进电机命令输入与输出.vi"("输入字符串"="S0/", "串口通信端口"=w849) -> ()  [unwired: 1 out]
                            }
                          }
                          n552 = Subtract(x=w839, y=w845) -> (x-y=w843:dbl)
                          n553 = Absolute Value(x=w843) -> (abs(x)=w842:dbl)
                          n554 = local read "精度"() -> (w846:dbl)
                          n555 = Less?(x=w842, y=w846) -> (x < y?=w847:bool)
                        }
                      }
                      frame True {
                        n556 = flat-sequence {
                          tunnel: [w857] -> _
                          tunnel: [w857] -> w854
                          tunnel: w852 -> [w857]
                          tunnel: [w855] -> w851
                          frame #0 {
                            n557 = property on="细分设置" class="DigNum (严格)"() -> ("Value"=w855:dbl)  [unwired: 2 in, 2 out]
                            n558 = Multiply(x=0.0, y=200.0) -> (x*y=w861:dbl)
                            n559 = Multiply(x=w861, y=w855) -> (x*y=w866:dbl)
                            n560 = Number To Fractional String(number=w866, precision (6)=i16 0 ("精度(6)")) -> (F-format string=w864:string)  [unwired: 2 out]
                            n561 = Concatenate Strings("Y=" ("字符串"), w864, "/" ("字符串")) -> (w859:string)
                            n562 = call "步进电机命令输入与输出.vi"("输入字符串"=w859, "串口通信端口"=w857) -> ()  [unwired: 1 out]
                            n563 = property on="等待时间" class="DigNum (严格)"() -> ("Value"=w856:u32)  [unwired: 2 in, 2 out]
                            n564 = Wait (ms)(milliseconds to wait=w856) -> ()  [unwired: 1 out]
                          }
                        }
                        n565 = while {
                          shift-right: [w868] -> w853
                          shift-left: w854 -> [w868]
                          shift-right: [w867] -> _
                          shift-left: w851 -> [w867]
                          stop <- w874 stop-if-true
                          n566 = property on="电机急停" class="Bool (严格)"() -> ("Value"=w875:bool)  [unwired: 2 in, 2 out]
                          n567 = call "X,Y,Z轴坐标查询.vi"("细分设置"=w867, "查询坐标轴"="Y", "串口通信端口"=w868) -> ("坐标(mm)"=w876:dbl)
                          n568 = case shown="真" w875 {
                            tunnel: w868 -> [_ w879]
                            frame False {
                            }
                            frame True {
                              n569 = call "步进电机命令输入与输出.vi"("输入字符串"="S0/", "串口通信端口"=w879) -> ()  [unwired: 1 out]
                            }
                          }
                          n570 = Multiply(x=w876, y=1.0 ("x")) -> (x*y=w872:dbl)
                          n571 = Subtract(x=w872, y=0.0 ("x")) -> (x-y=w870:dbl)
                          n572 = local read "精度"() -> (w873:dbl)
                          n573 = Absolute Value(x=w870) -> (abs(x)=w869:dbl)
                          n574 = property on="Y(mm)" class="DigNum (严格)"("Value"=w872) -> ()  [unwired: 2 in, 2 out]
                          n575 = Less?(x=w869, y=w873) -> (x < y?=w874:bool)
                        }
                      }
                    }
                    n576 = flat-sequence {
                      tunnel: w622 -> [w813]
                      tunnel: [w813] -> w621
                      frame #0 {
                        n577 = local read "毫秒计时值"() -> (w814:u32)
                        n578 = Tick Count (ms)() -> (millisecond timer value=w817:u32)
                        n579 = Subtract(x=w817, y=w814) -> (x-y=w815:u32)
                        n580 = Multiply(x=w815, y=0.001) -> (x*y=w818:dbl)
                        n581 = property on="已用时（s）" class="DigNum (严格)"("Value"=w818) -> ()  [unwired: 2 in, 2 out]
                      }
                    }
                  }
                  n582 = property on="已用时（s）" class="DigNum (严格)"("Visible"=TRUE ("可见")) -> ()  [unwired: 2 in, 2 out]
                  n583 = flat-sequence {
                    tunnel: w514 -> [w597]
                    tunnel: w513 -> [w598]
                    tunnel: [w598] -> w510
                    tunnel: [w597] -> w509
                    tunnel: [w600] -> w519
                    tunnel: w510 -> [w600]
                    tunnel: w509 -> [w601]
                    frame #0 {
                      n584 = property on="水平进度条" class="Slide (严格)"("Value"=u8 100 ("水平进度条")) -> ()  [unwired: 2 in, 2 out]
                    }
                    frame #1 {
                      n585 = local read "毫秒计时值"() -> (w605:u32)
                      n586 = property on="数组" class="Arr (严格)"("Value"=w601) -> ()  [unwired: 2 in, 2 out]
                      n587 = Transpose 2D Array(2D array=w601) -> (transposed array=w602:dbl[][])
                      n588 = Tick Count (ms)() -> (millisecond timer value=w606:u32)
                      n589 = property on="强度图" class="IntGraph (严格)"("Value"=w602) -> ()  [unwired: 2 in, 2 out]
                      n590 = Subtract(x=w606, y=w605) -> (x-y=w603:u32)
                      n591 = Multiply(x=w603, y=0.001) -> (x*y=w599:dbl)
                      n592 = property on="已用时（s）" class="DigNum (严格)"("Value"=w599) -> ()  [unwired: 2 in, 2 out]
                    }
                  }
                }
                event "分层图查看": Value Change {
                  n593 = event-data() -> ()  [unwired: 1 in, 6 out]
                  n594 = call "分层图显示1.2.1（导入色码表）.vi"("IN"=w882) -> ("OUT"=w881:string)  [unwired: 10 in]
                }
              }
            }
          }
        }
        n595 = dll-call lib="E:/PCI8552B/Driver/INF/Win32&Win64/amd64/PCI8552B_32.dll" fn="PCI8552B_StopDeviceAD" label="StopDeviceAD"("hDevice"="hDevice 2") -> ("hDevice"=w13:i32)  [unwired: 4 in, 2 out]
        n596 = dll-call lib="E:/PCI8552B/Driver/INF/Win32&Win64/amd64/PCI8552B_32.DLL" fn="PCI8552B_ReleaseDeviceAD" label="ReleaseDeviceAD"("hDevice"=w13) -> ("hDevice"=w12:i32)  [unwired: 4 in, 2 out]
        n597 = VISA Close(VISA resource name=w49) -> (error out=→"错误输出":errorcluster)  [unwired: 1 in]
        n598 = dll-call lib="E:/PCI8552B/Driver/INF/Win32&Win64/amd64/PCI8552B_32.DLL" fn="PCI8552B_ReleaseDevice" label="ReleaseDevice"("hDevice"=w12) -> ()  [unwired: 5 in, 2 out]
        "M_Length" <- w15
        "量程选择" <- w23
      }
    }
  }
  n599 = property on="高级设置" class="Bool"("Visible"=FALSE ("可见")) -> ()  [unwired: 2 in, 2 out]
  n600 = property on="定位模式" class="Bool"("Visible"=FALSE ("可见")) -> ()  [unwired: 2 in, 2 out]
  n601 = property on="已用时（s）" class="DigNum (严格)"("Visible"=FALSE ("可见")) -> ()  [unwired: 2 in, 2 out]
